vi "STP_22 - three_multiAO+dynamics.vi"() -> ()   [LabVIEW 2010]
uses:
  <vilib>/Math Plots/2D Math Plots/2D Compass/2D Compass XCtrl/2D Compass.xctl
  <vilib>/Platform/TimedLoop/XDataNode/nitl_modes.ctl
  <vilib>/Platform/TimedLoop/XDataNode/XDataNode.xnode
  <vilib>/Platform/TimedLoop/XDataNode/timing_clust.ctl
  <vilib>/Platform/TimedLoop/XDataNode/wakeup.ctl
  <vilib>/Utility/error.llb/DialogType.ctl
  <vilib>/DAQmx/write.llb/DAQmx Write (Analog 1D Wfm NChan NSamp).vi
  <vilib>/DAQmx/write.llb/DAQmx Write (Analog 2D DBL NChan NSamp).vi
  <vilib>/DAQmx/create/timing.llb/DAQmx Create Timing Source (Frequency).vi
  <vilib>/Instr/_visa.llb/VISA Configure Serial Port (Instr).vi
  <vilib>/Math Plots/2D Math Plots/2D Compass/2D Compass Datatype/Public/Plot Helper (Vector).vi
  <vilib>/DAQmx/create/channels.llb/DAQmx Create Channel (AO-Voltage-Basic).vi
  <vilib>/DAQmx/configure/timing.llb/DAQmx Timing (Sample Clock).vi
  <vilib>/daqmx/miscellaneous.llb/DAQmx Fill In Error Info.vi
  <vilib>/measure/matone.llb/Extract Single Tone Information 1 Chan.vi
  <vilib>/measure/NI_MABase.lvlib
  Program Files/National Instruments/LabVIEW 2010/resource/objmgr/daqmx.rc
  <vilib>/Platform/TimedLoop/XDataNode/XDNodeRunTimeDep.lvlib
  <vilib>/measure/NI_MAPro.lvlib
  <vilib>/Math Plots/2D Math Plots/2D Compass/2D Compass Datatype/2D Compass Datatype.lvclass
  <vilib>/Analysis/NI_AALBase.lvlib
  <vilib>/Analysis/NI_AALPro.lvlib
panel:
  out "rocof0":dbl[](array[numeric])
  out "rocof1":dbl[](array[numeric])
  out "ROCOF measured":dbl[](array[numeric])
  out "ROCOF reference":dbl[](array[numeric])
  out "Media":dbl
  in  "stop":bool
  out "Frequency reference":dbl[](array[numeric])
  out "Frequency measured":dbl[](array[numeric])
  out "Angle reference":dbl[](array[numeric])
  out "Angle measured":dbl[](array[numeric])
  out "Voltage reference":dbl[](array[numeric])
  out "Voltage measured":dbl[](array[numeric])
  out "freq1":dbl[](array[numeric])
  out "freq0":dbl[](array[numeric])
  out "magnitude1":dbl[](array[numeric])
  out "magnitude0":dbl[](array[numeric])
  in  "last amp":dbl
  out "phases0":dbl[](array[numeric])
  out "phases1":dbl[](array[numeric])
  out "initialized array":dbl[](array[numeric])
  out "Sine phase":dbl
  in  "Tab Control":T1(tab)
  out "Interf.\nAmplitude (%)":dbl
  out "Interf.\nFrequency (Hz)":dbl
  out "Amplitude (%)":dbl
  out "Harmonic order":i32
  out "reset\nphase?":bool
  out "Samples":dbl
  out "Frequency (Hz)":dbl
  out "Phase (deg)":dbl format="%.4f"
  out "Amplitude (V)":dbl format="%.4g"
  in  "Tab Control 3":T2(tab)
  in  "Interference":bool
  in  "Interf. Frequency":dbl caption="Frequency"
  in  "Interf. Amplitude":dbl caption="Amplitude (%)"
  in  "Amplitude (%)":dbl=10.0
  in  "Order":i32=2
  in  "Harmonics":bool
  in  "phase 2":dbl
  in  "duty cycle (%)":dbl=1.0
  in  "Pulse frequency":dbl=1.0
  in  "Noise":bool
  in  "Amplitude (rms)":dbl=0.0035355 format="%0.6f"
  in  "reset signal":bool
  in  "Phase":dbl format="%#.4f"
  in  "Frequency":dbl=50.0 format="%#.4f"
  in  "Offset":dbl=1.5 format="%#.4f"
  in  "Amplitude":dbl=5.0 format="%#.4f"
  in  "Seconds":dbl=100.0
  in  "Save without\nvariation":bool
  in  "Amp. (%) 4":dbl=10.0 caption="Amplitude (%)"
  in  "Frequency\ninterval 2":dbl=0.25 caption="Frequency\ninterval"
  in  "Final freq. 2":dbl=51.25 caption="Final freq."
  in  "Initial freq. 2":dbl=48.75 caption="Initial freq."
  in  "Interference\nauto variation":bool
  in  "Amp. (%) 3":dbl=10.0 caption="Amplitude (%)"
  in  "Order\ninterval":i32=1
  in  "Final order":i32=50
  in  "Initial order":i32=2
  in  "Harmonics\nauto variation":bool
  in  "Frequency\ninterval":dbl=0.1 format="%.4f"
  in  "Final freq.":dbl=55.0 format="%.4f"
  in  "Initial freq.":dbl=45.0 format="%.4f"
  in  "Freq. auto\nvariation":bool
  in  "Phase\ninterval":dbl=10.0 format="%.4f"
  in  "Final phase":dbl=180.0 format="%.4f"
  in  "Initial phase":dbl=-180.0 format="%.4f"
  in  "Phase auto\nvariation":bool
  in  "Amplitude\ninterval":dbl=0.1 format="%.4f"
  in  "Initial ampl.":dbl=0.5 format="%.4f"
  in  "Final ampl.":dbl=6.0 format="%.4f"
  in  "Ampl. auto\nvariation":bool
  in  "Boolean 2":bool
  in  "Dynamic tests?":bool
  in  "Final fmod":dbl=5.0
  in  "fmod interval":dbl=0.2
  in  "Initial fmod":dbl
  in  "Modulation\nauto variation":bool
  in  "fmod":dbl
  out "fmod (Hz)":dbl
  in  "kx":dbl=0.1
  in  "Enum":T3(ring)
  in  "ka":dbl=0.1
  in  "Freq. Ramp":bool
  in  "Signal generation":bool=TRUE
  in  "File name":path=path "teste.txt"
  in  "Data save":bool
  in  "Boolean":bool
  in  "step time":i32=2
  out "step?":bool
  out "Cycle visualization":dbl[](graph)
  in  "Boolean 3":bool
  out "Phasors visualization":refnum<class "2D Plot Datatype.lvclass">[](xcontrol) caption="2D Compass"
  in  "Porta":refnum<visa-resource-name>="COM5"
  in  "baud rate (kB)":u32=115200
  in  "data bits (8)":u16=8
  in  "timeout (ms)":u32=5000
  in  "parity (0:none)":enum16{"None", "Odd", "Even", "Mark", "Space"}(ring)
  in  "flow control (0:none)":u16(ring) items=["None", "XON/XOFF", "RTS/CTS", "XON/XOFF & RTS/CTS", "DTR/DSR", "XON/XOFF & DTR/DSR"]
  in  "stop bits (10: 1 bit)":u16(ring)=10 items=["1.0"=10, "1.5"=15, "2.0"=20]
  in  "Serial communication":bool=TRUE
  in  "Interference 2":bool caption="Interference"
  in  "amplitude":dbl=1.0 caption="Amp. (%)" format="%#.4p"
  in  "Interf. Frequency 2":dbl=10.0 caption="Frequency (Hz)"
  in  "Harmonics 2":bool caption="Harmonics"
  in  "Amp. (%) 2":dbl caption="Amp. (%)"
  in  "Order 2":i32=2 caption="Order"
  out "Frequency":dbl
  in  "Offset 2":dbl=1.5 caption="Offset"
  out "Phase (degrees) 2":dbl caption="Phase (°)" format="%.4f"
  in  "Amplitude 2":dbl=1.3 caption="Amplitude"
  in  "Frequency 2":dbl=60.0 caption="Frequency"
  in  "Phase 2":dbl caption="Phase"
  in  "reset signal 2":bool caption="reset\nsignal"
  in  "Frequency\noff-set":dbl
  in  "Magnitude\noff-set":dbl
  in  "Magnitude\ncoefficient":dbl=1.0
  in  "Angle\noff-set":dbl
  out "mean rocof":dbl caption="ROCOF (Hz/s)" format="%.8g"
  out "max rocof":dbl caption="ROCOF (Hz/s)" format="%.8g"
  out "mean freq":dbl caption="Frequency (Hz)" format="%.8g"
  out "mean tve":dbl caption="TVE (%)" format="%.8g"
  out "mean phase":dbl caption="Phase (º)" format="%.8g"
  out "mean dev":dbl caption="Magnitude (%)" format="%.8g"
  out "max magnitude":dbl caption="Magnitude (%)" format="%.8g"
  out "max tve":dbl caption="TVE (%)" format="%.8g"
  out "max freq":dbl caption="Frequency (Hz)" format="%.8g"
  out "max phase":dbl caption="Phase (º)" format="%.8g"
  in  "Tab Control 2":T4(tab)
  out "Magnitude measures (V)":dbl[][](graph)
  in  "?":bool
  out "Phase measures (º)":dbl[][](graph)
  in  "?":bool
  in  "Fase ref":enum16{"R", "S", "T"}(ring)
  out "Frequency measures (Hz)":dbl[][](graph)
  in  "?":bool
  out "ROCOF (Hz/s)":dbl[][](graph)
  in  "?":bool
  in  "?":bool
  out "Phase measures (º) 2":dbl[](graph)
  out "Iteration Duration 2":i64
  out "Finished Late? [i-1]":bool
  out "Iteration Duration":i64
  out "Iteration Duration 3":i64
  # "Synchrophasors Test Platform"
  # "A real-time platform for PMU development."
  # "Actual generation"
  # "PPS parameters"
  # "Noise"
  # "Sinusoid parameters"
  # "Max errors:"
  # "Mean errors:"
  # "Signal generation parameters:"
  # "On-line corrections (received data):"
  # "This is a project developed by Flavio Lori Grando, during Masters in Electrical Engineering Graduate Program (PPGEE) of Federal University of Technology - Paraná, Brazil.\n\nContact: flavio.grando.eng@gmail.com"
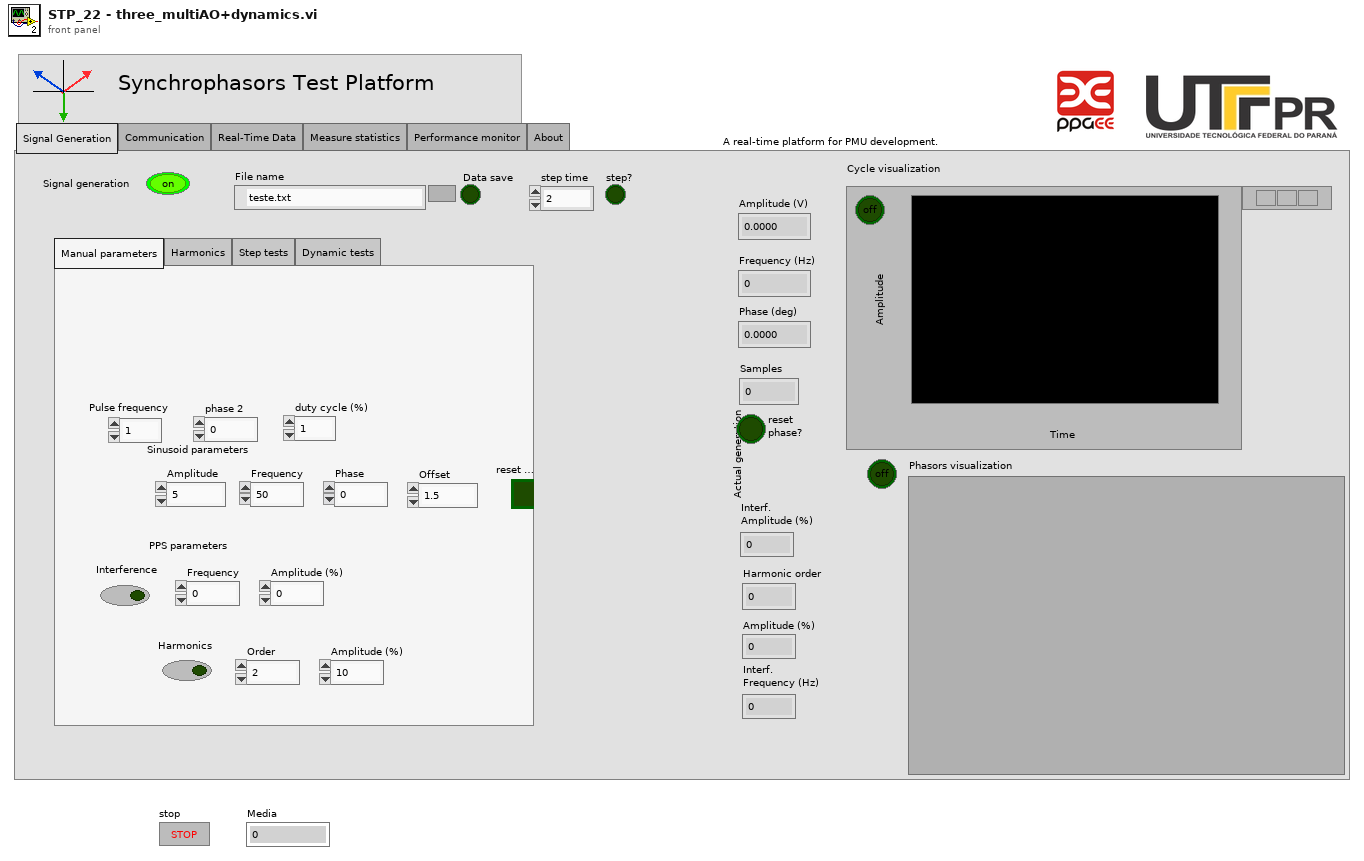
[diagram p1: front panel]
types:
  T1 = enum32{"Signal Generation", "Communication", "Real-Time Data", "Measure statistics", "Performance monitor", "About"}
  T2 = enum32{"Manual parameters", "Harmonics", "Step tests", "Dynamic tests"}
  T3 = enum16{"Amplitude modulation", "Phase modulation", "Frequency ramp", "Frequency ramp 2", "Frequency ramp 3", "Frequency ramp 4", "Frequency ramp 5", "Frequency ramp 6"}
  T4 = enum32{"Magnitude", "Phase", "Frequency", "ROCOF", "Phase deviation"}
  T5 = enum16{"Sine Wave", "Triangle Wave", "Square Wave", "Sawtooth Wave"}
  T6 = typedef "XDNodeRunTimeDep.lvlib/nitl_modes.ctl" = enum32{"No Change", "Process missed periods, maintain original phase", "Discard missed periods, maintain original phase", "Process missed periods, ignore original phase", "Discard missed periods, ignore original phase"}
  T7 = cluster{"frequency":dbl, "amplitude":dbl, "phase":dbl}[]
  T8 = typedef "XDNodeRunTimeDep.lvlib/timing_clust.ctl" = cluster{"Expected End [f-1]":u64, "Actual End [f-1]":u64, "Finished Late? [f-1]":bool, "Expected End [i-1]":u64, "Actual End [i-1]":u64, "Finished Late? [i-1]":bool, "Expected Start [i]":u64, "Actual Start [i]":u64, "Expected Start [f]":u64, "Actual Start [f]":u64, "Source Name":string, "Structure Name":string, "Period":i64, "Deadline":i64, "Offset":i64, "Start":i64, "Priority":i32, "Timeout":i32, "Mode":T6, "Wakeup Reason":T9, "Error":errorcluster, "Source Type":string, "Secondary Source Type":string, "Global End Time":u64, "Global Start Time":u64, "Frame Duration":u64, "Iteration Duration":u64, "Assigned CPU":i32, "I/O Scan Engine Mode":u32}
  T9 = typedef "XDNodeRunTimeDep.lvlib/wakeup.ctl" = enum32{"Normal", "Aborted", "Asynchronous wakeup", "Timing source error", "Timed loop error", "Timeout"}
  T10 = typedef "DialogType.ctl" = u16
  T11 = enum16{"open", "replace", "create", "open or create", "replace or create", "replace or create with confirmation"}
  T12 = cluster{"max ref":dbl, "min ref":dbl, "mean ref":dbl, "max dev":dbl, "min dev":dbl, "mean dev":dbl, "max meas":dbl, "min meas":dbl, "mean meas":dbl}
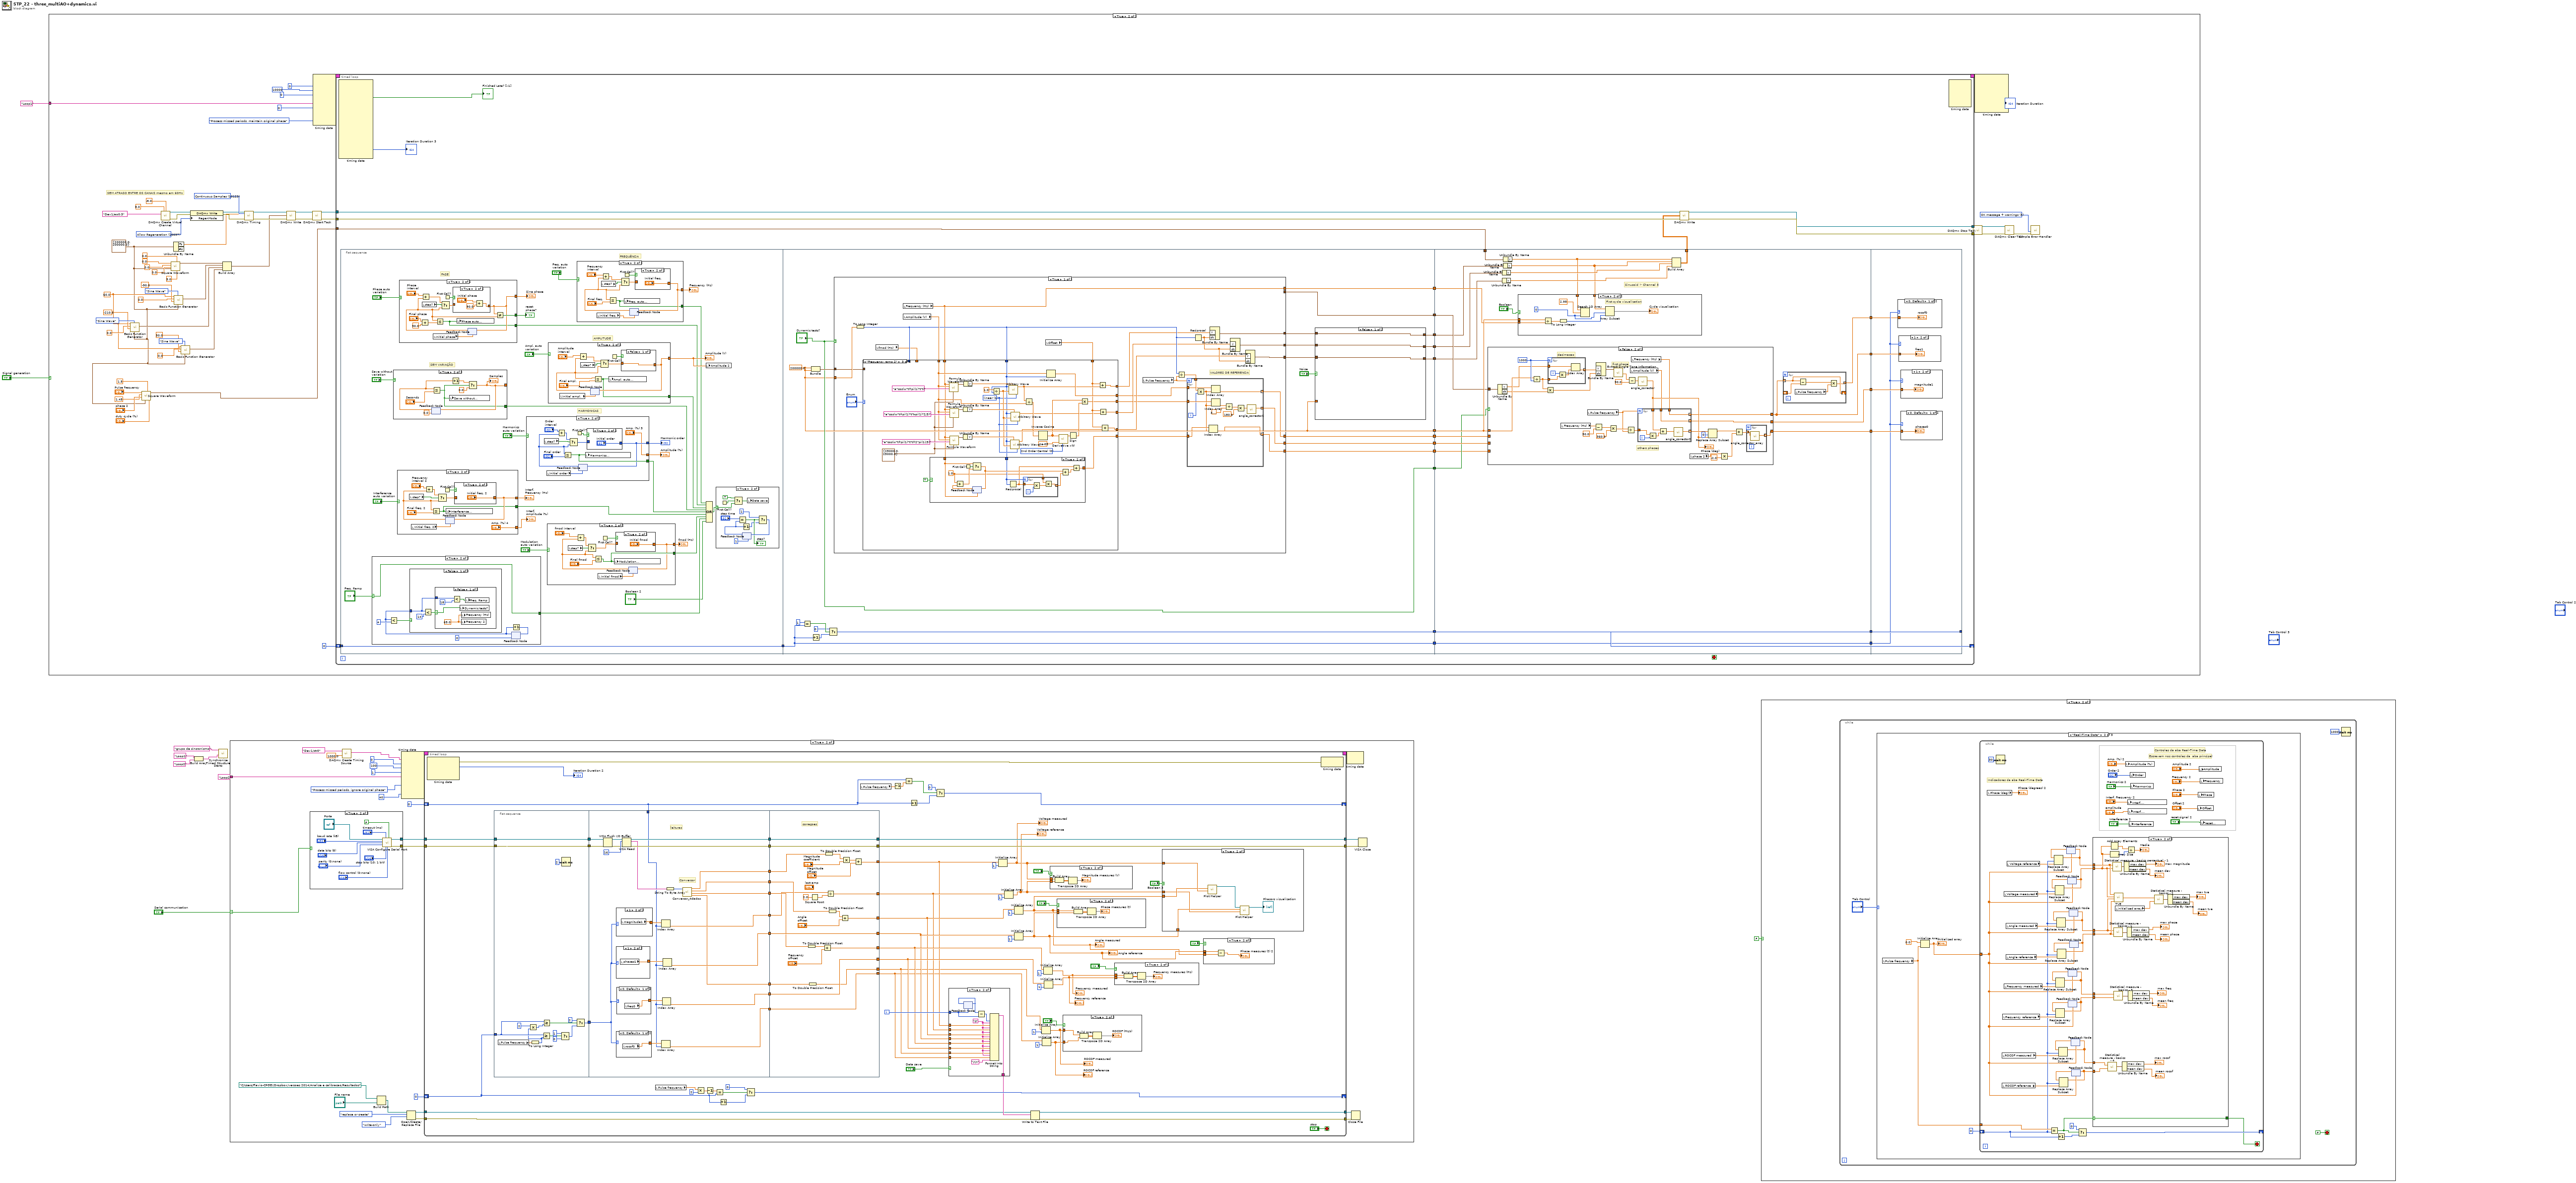
[diagram p0: block diagram]
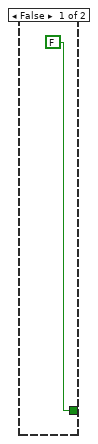
[diagram p4: hidden frame]
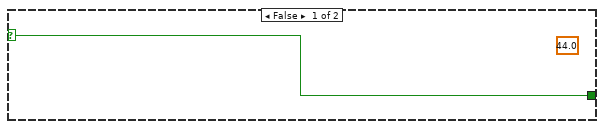
[diagram p7: hidden frame]
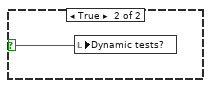
[diagram p8: hidden frame]
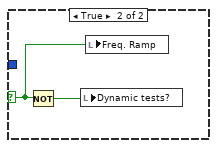
[diagram p9: hidden frame]
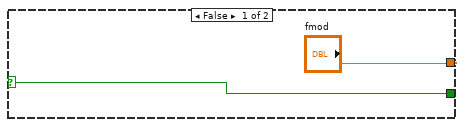
[diagram p10: hidden frame]
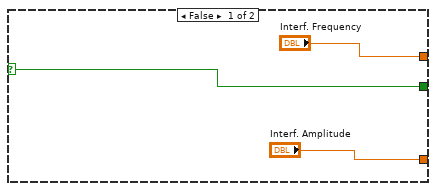
[diagram p12: hidden frame]
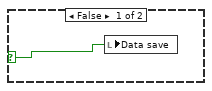
[diagram p14: hidden frame]
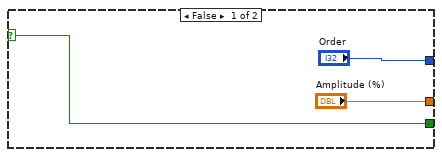
[diagram p15: hidden frame]
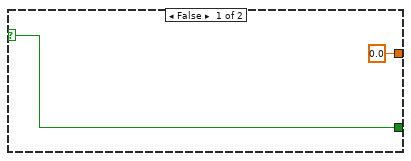
[diagram p17: hidden frame]
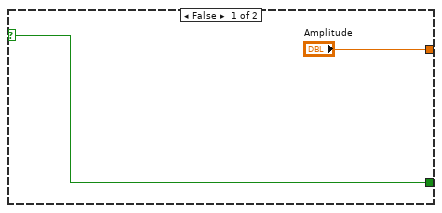
[diagram p18: hidden frame]
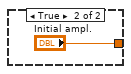
[diagram p19: hidden frame]
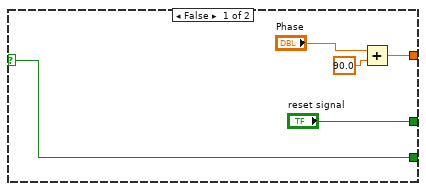
[diagram p20: hidden frame]
diagram:
  n1 = case shown="True" "Signal generation" {
    tunnel: "Loop1" -> [_ w32]
    frame False {
    }
    frame True {
      w19 = 60.0 ("frequency")
      w60 = 10097 items=["Allow Regeneration"=10097, "Do Not Allow Regeneration"=10158] ("RegenMode")
      w13 = cluster{"Fs":dbl, "#s":dbl} {"Fs"=200000.0, "#s"=200000.0} ("Continuous buffer")
      w63 = 10123 items=["Finite Samples"=10178, "Continuous Samples"=10123] ("sample mode")
      w64 = T10 3 items=["no dialog", "OK message", "continue or stop message", "OK message + warnings", "continue/stop + warnings"] ("type of dialog (OK msg:1)")
      # "SEM ATRASO ENTRE OS CANAIS mesmo em 60Hz"
      n2 = call <vilib>:"Basic Function Generator.vi"("sampling info"=w13, "signal type"=T5."Sine Wave" ("signal type 4"), "phase"=-210.0 ("offset 4"), "amplitude"=0.0 ("amplitude 3"), "frequency"=w19) -> ("signal out"=w24:waveform(dbl))  [unwired: 4 in, 2 out]
      n3 = call <vilib>:"Square Waveform.vi"("duty cycle (%)"="duty cycle (%)", "offset"=1.5, "sampling info"=w13, "phase"="phase 2", "amplitude"=1.45, "frequency"="Pulse frequency") -> ("signal out"=w28:waveform(dbl))  [unwired: 4 in, 1 out]
      n4 = call-poly <vilib>:"DAQmx Create Virtual Channel.vi"("maximum value"=8.0 ("Maximum Value"), "minimum value"=-8.0 ("Minimum Value"), "physical channels"=tag "Dev1/ao0:3" ("Physical Channel")) -> ("task out"=w39:refnum<k21>, "error out"=w40:errorcluster)  [unwired: 11 in]
      n5 = call <vilib>:"Square Waveform.vi"("duty cycle (%)"=5.0, "offset"=0.0, "sampling info"=w13, "phase"=0.0, "amplitude"=0.0, "frequency"=0.0) -> ("signal out"=w30:waveform(dbl))  [unwired: 4 in, 1 out]
      n6 = Unbundle By Name(w13) -> ("Fs"=w11:dbl)  [unwired: 1 out]
      n7 = call <vilib>:"Basic Function Generator.vi"("sampling info"=w13, "signal type"=T5."Sine Wave" ("signal type 4"), "phase"=-90.0 ("offset 4"), "amplitude"=0.0 ("amplitude 3"), "frequency"=w19) -> ("signal out"=w31:waveform(dbl))  [unwired: 4 in, 2 out]
      n8 = call <vilib>:"Basic Function Generator.vi"("sampling info"=w13, "signal type"=T5."Sine Wave" ("signal type 4"), "phase"=30.0 ("offset 4"), "amplitude"=0.0 ("amplitude 3"), "frequency"=w19) -> ("signal out"=w20:waveform(dbl))  [unwired: 4 in, 2 out]
      n9 = property class="DAQmx Write"(reference=w39, error in=w40, "RegenMode"=w60) -> (reference out=w12:refnum<k21>, error out=w61:errorcluster)
      n10 = Build Array(w30, w31, w24, w20) -> (w33:waveform(dbl)[])
      n11 = call-poly <vilib>:"DAQmx Timing.vi"("task/channels in"=w12, "sample mode"=w63, "rate"=w11, "error in"=w61) -> ("task out"=w35:refnum<k21>, "error out"=w34:errorcluster)  [unwired: 10 in]
      n12 = call-poly <vilib>:"DAQmx Write.vi"("task/channels in"=w35, "data"=w33, "error in"=w34) -> ("task out"=w44:refnum<k21>, "error out"=w45:errorcluster)  [unwired: 10 in, 1 out]
      n13 = call <vilib>:"DAQmx Start Task.vi"("task/channels in"=w44, "error in"=w45) -> ("task out"=w36:refnum<k21>, "error out"=w37:errorcluster)  [unwired: 12 in]
      n14 = node-c288(i64 0 ("Period"), 10000 ("Priority"), 0 ("Processor"), w32, i64 0 ("Deadline"), nitl_modes."Process missed periods, maintain original phase" ("Mode")) -> (w68:T8)  [unwired: 4 in]
      n15 = timed-loop {
        tunnel: w36 -> [w72]
        tunnel: [w89] -> w53
        tunnel: [w88] -> w52
        timing: w68 -> [_]
        timing-out: [_] -> w67
        shift-right: [w96] -> _
        shift-left: 0 -> [w76]
        tunnel: w37 -> [w90]
        tunnel: w28 -> [w71]
        stop <- _ stop-if-true
        n16 = node-c288() -> (→"Finished Late? [i-1]":bool, →"Iteration Duration 3":i64)  [unwired: 1 in, 15 out]
        n17 = flat-sequence {
          tunnel: w76 -> [w120]
          tunnel: [w120] -> w86
          tunnel: [w275] -> w87
          tunnel: w86 -> [w274]
          tunnel: [w274] -> w85
          tunnel: [w261] -> w84
          tunnel: [w280] -> w83
          tunnel: [w270] -> w81
          tunnel: [w269] -> w80
          tunnel: [w271] -> w79
          tunnel: [w273] -> w78
          tunnel: [w265] -> w75
          tunnel: [w263] -> w74
          tunnel: [w264] -> w73
          tunnel: ["Dynamic tests?"] -> w69
          tunnel: [w679] -> w95
          tunnel: [w677] -> w94
          tunnel: [w670] -> w93
          tunnel: [w658] -> w92
          tunnel: w87 -> [w679]
          tunnel: w85 -> [w678]
          tunnel: [w678] -> w91
          tunnel: [w674] -> w70
          tunnel: w84 -> [w676]
          tunnel: w83 -> [w675]
          tunnel: [w657] -> w82
          tunnel: w81 -> [w669]
          tunnel: w80 -> [w668]
          tunnel: w79 -> [w663]
          tunnel: w78 -> [w673]
          tunnel: w75 -> [w672]
          tunnel: w74 -> [w659]
          tunnel: w73 -> [w671]
          tunnel: w71 -> [w662]
          tunnel: w69 -> [w660]
          tunnel: w95 -> [w749]
          tunnel: [w749] -> w96
          tunnel: w94 -> [w748]
          tunnel: w93 -> [w747]
          tunnel: w92 -> [w746]
          tunnel: w91 -> [w745]
          tunnel: w82 -> [w744]
          frame #0 {
            # "HARMONICAS"
            # "SEM VARIA敲O"
            # "FASE"
            # "FREQUÊNCIA"
            # "AMPLITUDE"
            n18 = case shown="True" "Freq. Ramp" {
              selector: "Freq. Ramp" -> [w126 w127]
              tunnel: [w126 w127] -> w99
              frame False {
                (unwired) 44.0 ("Initial freq. 3")
              }
              frame True {
                n19 = feedback #1(0) -> (w129:i32)
                n20 = Less?(x=w129, y=4) -> (x < y?=w128:bool)
                n21 = case shown="False" w128 {
                  selector: w128 -> [_ w142]
                  tunnel: w129 -> [w134 _]
                  frame False {
                    n22 = Less?(x=w134, y=14) -> (x < y?=w133:bool)
                    n23 = case shown="False" w133 {
                      selector: w133 -> [w136 w141]
                      tunnel: w134 -> [w139 _]
                      frame False {
                        w137 = 65.0 ("Frequency")
                        n24 = Less?(x=w139, y=18) -> (x < y?=w138:bool)
                        n25 = local write "Dynamic tests?"(w136) -> ()
                        n26 = local write "Frequency (Hz)"(w137) -> ()
                        n27 = local write "Frequency 2"(w137) -> ()
                        n28 = local write "Freq. Ramp"(w138) -> ()
                      }
                      frame True {
                        n29 = local write "Dynamic tests?"(w141) -> ()
                      }
                    }
                  }
                  frame True {
                    n30 = Not(x=w142) -> (.not. x?=w143:bool)
                    n31 = local write "Dynamic tests?"(w143) -> ()
                    n32 = local write "Freq. Ramp"(w142) -> ()
                  }
                }
                n33 = Increment(x=w129) -> (x+1=w131:i32)
                n34 = feedback-in #1(w131) -> ()
              }
            }
            n35 = case shown="True" "Save without\nvariation" {
              selector: "Save without\nvariation" -> [w202 _]
              tunnel: [0.0 ("f") w205] -> _
              tunnel: [w202 w204] -> w114
              frame False {
              }
              frame True {
                n36 = feedback #2(0.0 ("f")) -> (w207:dbl)
                n37 = Less Or Equal?(x=w207, y="Seconds") -> (x <= y?=w204:bool)
                n38 = local write "Save without\nvariation"(w204) -> ()
                n39 = Increment(x=w207) -> (x+1=w209:dbl)
                n40 = Select(t=w209, s=w204, f=0.0) -> (s? t:f=w205:dbl)
                "Samples" <- w205
                n41 = feedback-in #2(w205) -> ()
              }
            }
            n42 = case shown="True" "Interference\nauto variation" {
              selector: "Interference\nauto variation" -> [w158 _]
              tunnel: ["Interf. Frequency" w167] -> w106
              tunnel: ["Interf. Amplitude" "Amp. (%) 4"] -> w105
              tunnel: [w158 w161] -> w104
              frame False {
              }
              frame True {
                n43 = local read "step?"() -> (w164:bool)
                n44 = local read "Initial freq. 2"() -> (w168:dbl)
                n45 = First Call?() -> (First Call?: T/F=w171:bool)
                n46 = feedback #3(w168) -> (w163:dbl)
                n47 = Add(x="Frequency\ninterval 2", y=w163) -> (x+y=w165:dbl)
                n48 = Less Or Equal?(x=w163, y="Final freq. 2") -> (x <= y?=w161:bool)
                n49 = Select(t=w165, s=w164, f=w163) -> (s? t:f=w170:dbl)
                n50 = local write "Interference\nauto variation"(w161) -> ()
                n51 = case shown="True" w171 {
                  tunnel: [w172 "Initial freq. 2"] -> w167
                  tunnel: w170 -> [w172 _]
                  frame False {
                  }
                  frame True {
                  }
                }
                n52 = feedback-in #3(w167) -> ()
              }
            }
            "Interf.\nFrequency (Hz)" <- w106
            "Interf.\nAmplitude (%)" <- w105
            n53 = case shown="True" "Phase auto\nvariation" {
              selector: "Phase auto\nvariation" -> [w225 _]
              tunnel: ["reset signal" w240] -> w125
              tunnel: [w227 w239] -> w115
              tunnel: [w225 w234] -> w112
              frame False {
                n54 = Add(x="Phase", y=90.0) -> (x+y=w227:dbl)
              }
              frame True {
                n55 = Add(x="Final phase", y=90.0) -> (x+y=w236:dbl)
                n56 = local read "step?"() -> (w230:bool)
                n57 = local read "Initial phase"() -> (w238:dbl)
                n58 = First Call?() -> (First Call?: T/F=w241:bool)
                n59 = feedback #4(w238) -> (w232:dbl)
                n60 = Add(x="Phase\ninterval", y=w232) -> (x+y=w231:dbl)
                n61 = Less Or Equal?(x=w232, y=w236) -> (x <= y?=w234:bool)
                n62 = Select(t=w231, s=w230, f=w232) -> (s? t:f=w233:dbl)
                n63 = case shown="True" w241 {
                  tunnel: [w243 w244] -> w239
                  tunnel: w233 -> [w243 _]
                  frame False {
                  }
                  frame True {
                    n64 = Add(x="Initial phase", y=90.0) -> (x+y=w244:dbl)
                  }
                }
                n65 = local write "Phase auto\nvariation"(w234) -> ()
                n66 = feedback-in #4(w239) -> ()
                n67 = Not Equal?(x=w239, y=w232) -> (x != y?=w240:bool)
              }
            }
            "Sine phase" <- w115
            "reset\nphase?" <- w125
            n68 = case shown="True" "Harmonics\nauto variation" {
              selector: "Harmonics\nauto variation" -> [w187 _]
              tunnel: ["Order" w193] -> w110
              tunnel: [w187 w194] -> w108
              tunnel: ["Amplitude (%)" "Amp. (%) 3"] -> w109
              frame False {
              }
              frame True {
                n69 = local read "step?"() -> (w196:bool)
                n70 = local read "Initial order"() -> (w198:i32)
                n71 = First Call?() -> (First Call?: T/F=w195:bool)
                n72 = feedback #5(w198) -> (w191:i32)
                n73 = Add(x="Order\ninterval", y=w191) -> (x+y=w190:i32)
                n74 = Less Or Equal?(x=w191, y="Final order") -> (x <= y?=w194:bool)
                n75 = Select(t=w190, s=w196, f=w191) -> (s? t:f=w199:i32)
                n76 = local write "Harmonics\nauto variation"(w194) -> ()
                n77 = case shown="True" w195 {
                  tunnel: [w200 "Initial order"] -> w193
                  tunnel: w199 -> [w200 _]
                  frame False {
                  }
                  frame True {
                  }
                }
                n78 = feedback-in #5(w193) -> ()
              }
            }
            "Harmonic order" <- w110
            "Amplitude (%)" <- w109
            n79 = case shown="True" "Modulation\nauto variation" {
              selector: "Modulation\nauto variation" -> [w145 _]
              tunnel: [w145 w148] -> w102
              tunnel: ["fmod" w147] -> w101
              frame False {
              }
              frame True {
                n80 = local read "step?"() -> (w154:bool)
                n81 = local read "Initial fmod"() -> (w146:dbl)
                n82 = First Call?() -> (First Call?: T/F=w155:bool)
                n83 = feedback #6(w146) -> (w151:dbl)
                n84 = Add(x="fmod interval", y=w151) -> (x+y=w153:dbl)
                n85 = Select(t=w153, s=w154, f=w151) -> (s? t:f=w149:dbl)
                n86 = Less Or Equal?(x=w151, y="Final fmod") -> (x <= y?=w148:bool)
                n87 = local write "Modulation\nauto variation"(w148) -> ()
                n88 = case shown="True" w155 {
                  tunnel: [w156 "Initial fmod"] -> w147
                  tunnel: w149 -> [w156 _]
                  frame False {
                  }
                  frame True {
                  }
                }
                n89 = feedback-in #6(w147) -> ()
              }
            }
            "fmod (Hz)" <- w101
            n90 = case shown="True" "Ampl. auto\nvariation" {
              selector: "Ampl. auto\nvariation" -> [w211 _]
              tunnel: ["Amplitude" w220] -> w119
              tunnel: [w211 w215] -> w113
              frame False {
              }
              frame True {
                n91 = local read "Initial ampl."() -> (w219:dbl)
                n92 = local read "step?"() -> (w216:bool)
                n93 = feedback #7(w219) -> (w214:dbl)
                n94 = Add(x="Amplitude\ninterval", y=w214) -> (x+y=w218:dbl)
                n95 = Less Or Equal?(x=w214, y="Final ampl.") -> (x <= y?=w215:bool)
                n96 = Select(t=w218, s=w216, f=w214) -> (s? t:f=w217:dbl)
                n97 = local write "Ampl. auto\nvariation"(w215) -> ()
                n98 = First Call?() -> (First Call?: T/F=w221:bool)
                n99 = case shown="False" w221 {
                  tunnel: [w223 "Initial ampl."] -> w220
                  tunnel: w217 -> [w223 _]
                  frame False {
                  }
                  frame True {
                  }
                }
                n100 = feedback-in #7(w220) -> ()
              }
            }
            "Amplitude (V)" <- w119
            n101 = case shown="True" "Freq. auto\nvariation" {
              selector: "Freq. auto\nvariation" -> [w248 _]
              tunnel: ["Frequency" w255] -> w117
              tunnel: [w248 w253] -> w111
              frame False {
              }
              frame True {
                n102 = local read "Initial freq."() -> (w254:dbl)
                n103 = local read "step?"() -> (w249:bool)
                n104 = First Call?() -> (First Call?: T/F=w257:bool)
                n105 = feedback #8(w254) -> (w250:dbl)
                n106 = Add(x="Frequency\ninterval", y=w250) -> (x+y=w251:dbl)
                n107 = Less Or Equal?(x=w250, y="Final freq.") -> (x <= y?=w253:bool)
                n108 = Select(t=w251, s=w249, f=w250) -> (s? t:f=w252:dbl)
                n109 = local write "Freq. auto\nvariation"(w253) -> ()
                n110 = case shown="True" w257 {
                  tunnel: [w259 "Initial freq."] -> w255
                  tunnel: w252 -> [w259 _]
                  frame False {
                  }
                  frame True {
                  }
                }
                n111 = feedback-in #8(w255) -> ()
              }
            }
            "Frequency (Hz)" <- w117
            n112 = local write "Amplitude 2"(w119) -> ()
            n113 = Compound Arithmetic op=OR(w111, w112, w113, w114, w108, w104, w102, w99, "Boolean 2") -> (w116:bool)
            n114 = case shown="True" w116 {
              selector: w116 -> [w174 w183]
              frame False {
                n115 = local write "Data save"(w174) -> ()
              }
              frame True {
                n116 = First Call?() -> (First Call?: T/F=w185:bool)
                n117 = Select(t=TRUE, s=w185, f=w183) -> (s? t:f=w182:bool)
                n118 = feedback #9(1 ("f")) -> (w175:i32)
                n119 = Equal?(x="step time", y=w175) -> (x = y?=w178:bool)
                "step?" <- w178
                n120 = Increment(x=w175) -> (x+1=w176:i32)
                n121 = local write "Data save"(w182) -> ()
                n122 = Select(t=1 ("f"), s=w178, f=w176) -> (s? t:f=w181:i32)
                n123 = feedback-in #9(w181) -> ()
              }
            }
          }
          frame #1 {
            w261 = 200000.0 ("#s")
            n124 = Equal?(x=1, y=w274) -> (x = y?=w279:bool)
            n125 = Bundle("#s"=w261, "#s"=w261) -> (w281:cluster{"#s":dbl, "#s":dbl})  [unwired: 1 in]
            n126 = Increment(x=w274) -> (x+1=w277:i32)
            n127 = Select(t=0, s=w279, f=w277) -> (s? t:f=w275:i32)
            n128 = case shown="True" "Dynamic tests?" {
              tunnel: w281 -> [w305 w601]
              tunnel: [w309 w603] -> w280
              tunnel: [w314 w595] -> w272
              tunnel: [w313 w594] -> w268
              tunnel: [w319 w590] -> w266
              tunnel: [_ w585] -> w273
              tunnel: w261 -> [w317 _]
              tunnel: [w308 _] -> w265
              tunnel: [w307 _] -> w264
              tunnel: [w298 _] -> w263
              frame True {
                # "VALORES DE REFERENCIA"
                n129 = To Long Integer(number=w317) -> (32bit integer=w311:i32)
                n130 = local read "fmod (Hz)"() -> (w306:dbl)
                n131 = local read "Frequency (Hz)"() -> (w309:dbl)
                n132 = local read "Amplitude (V)"() -> (w318:dbl)
                n133 = local read "Offset"() -> (w297:dbl)
                n134 = case shown="\"Frequency ramp 2\"" "Enum" {
                  tunnel: w318 -> [w331 w367 w425 w487 w500 _ w512 w559]
                  tunnel: w309 -> [w328 _ w423 w478 _ _ w514 w545]
                  tunnel: w311 -> [_ w374 w428 _ _ _ w513 w538]
                  tunnel: [w345 w381 w414 w481 _ _ w506 w554] -> w299
                  tunnel: [w325 w382 w420 w488 w498 _ w504 w536] -> w302
                  tunnel: [w323 w380 w415 w488 w497 _ w523 w547] -> w304
                  tunnel: [w322 w379 w417 w488 w496 _ w522 w546] -> w303
                  tunnel: w311 -> [w327 w375 _ w485 w495 _ _ w534]
                  tunnel: [w339 w372 w427 w483 _ _ w503 w544] -> w300
                  tunnel: w306 -> [w337 _ _ _ _ _ _ w539]
                  tunnel: w305 -> [w338 _ _ w489 _ _ _ w537]
                  tunnel: [w330 _ w431 _ _ _ w511 w536] -> w301
                  tunnel: w297 -> [w321 _ w419 _ _ _ _ _]
                  frame "Phase modulation" {
                    # "referencia"
                    n135 = call <vilib>:"Sine Waveform.vi"("sampling info"=w338, "phase"=-90.0, "amplitude"="ka", "frequency"=w337) -> ("signal out"=w341:waveform(dbl))  [unwired: 6 in, 1 out]
                    n136 = call <vilib>:"Sine Waveform.vi"("sampling info"=w338, "phase"=-180.0, "amplitude"="ka", "frequency"=w337) -> ("signal out"=w335:waveform(dbl))  [unwired: 6 in, 1 out]
                    n137 = Unbundle By Name(w341) -> ("Y"=w332:dbl[])
                    n138 = Unbundle By Name(w335) -> ("Y"=w334:dbl[])
                    n139 = Reciprocal(x=w327) -> (1/x=w329:dbl)
                    n140 = Multiply(x=w328, y=6.283185307179586) -> (x*y=w343:dbl)
                    n141 = Divide(x=6.283185307179586, y=3.0) -> (x/y=w348:dbl)
                    n142 = Multiply(x=w343, y=w329) -> (x*y=w344:dbl)
                    n143 = for {
                      N: w327 -> [_]
                      tunnel: w344 -> [w356]
                      tunnel: [w364] -> w351 mode=indexing
                      tunnel: [w353] -> w345 mode=indexing
                      tunnel: w348 -> [w361]
                      tunnel: [w360] -> w347 mode=indexing
                      tunnel: [w359] -> w346 mode=indexing
                      tunnel: w332 -> [w353] mode=indexing
                      tunnel: [w354] -> w330 mode=indexing
                      tunnel: w331 -> [w354]
                      i -> [w355]
                      n144 = Multiply(x=w356, y=w355) -> (x*y=w358:dbl)
                      n145 = Add(x=w358, y=w353) -> (x+y=w357:dbl)
                      n146 = Add(x=w357, y=w361) -> (x+y=w362:dbl)
                      n147 = Subtract(x=w357, y=w361) -> (x-y=w363:dbl)
                      n148 = Cosine(x=w362) -> (cos(x)=w360:dbl)
                      n149 = Cosine(x=w363) -> (cos(x)=w359:dbl)
                      n150 = Cosine(x=w357) -> (cos(x)=w364:dbl)
                    }
                    n151 = Multiply(x=w334, y=w337) -> (x*y=w340:dbl[])
                    n152 = Multiply(x=w331, y=w346) -> (x*y=w324:dbl[])
                    n153 = Multiply(x=w331, y=w347) -> (x*y=w320:dbl[])
                    n154 = Multiply(x=w331, y=w351) -> (x*y=w326:dbl[])
                    n155 = Subtract(x=w328, y=w340) -> (x-y=w339:dbl[])
                    n156 = Add(x=w321, y=w326) -> (x+y=w325:dbl[])
                    n157 = Add(x=w321, y=w320) -> (x+y=w322:dbl[])
                    n158 = Add(x=w321, y=w324) -> (x+y=w323:dbl[])
                  }
                  frame "Frequency ramp" {
                    w366 = 6.283185307179586
                    n159 = Bundle("#s"=50000.0, "#s"=500000.0) -> (w370:cluster{"#s":dbl, "#s":dbl})  [unwired: 1 in]
                    n160 = case shown="False" FALSE {
                      tunnel: [w397 w401] -> w368
                      tunnel: w375 -> [w393 _]
                      tunnel: w370 -> [_ w399]
                      frame False {
                        n161 = Divide(x=0.5 ("samples"), y=w393) -> (x/y=w396:dbl)
                        n162 = call <vilib>:"Sawtooth Wave.vi"("samples"=w393, "frequency"=w396, "reset phase"=FALSE) -> ("sawtooth wave"=w394:dbl[])  [unwired: 2 in, 2 out]
                        n163 = Negate(x=w394) -> (-x=w397:dbl[])
                      }
                      frame True {
                        n164 = call <vilib>:"Sawtooth Waveform.vi"("sampling info"=w399, "reset signal"=TRUE, "frequency"=0.5) -> ("signal out"=w402:waveform(dbl))  [unwired: 7 in, 1 out]
                        n165 = Unbundle By Name(w402) -> ("Y"=w401:dbl[])
                      }
                    }
                    n166 = Multiply(x=w366, y=w366) -> (x*y=w390:dbl)
                    n167 = Multiply(x=w368, y=3.141592653589793) -> (x*y=w377:dbl[])
                    n168 = Divide(x=6.283185307179586, y=3.0) -> (x/y=w385:dbl)
                    n169 = Multiply(x=w390, y=1e-05) -> (x*y=w389:dbl)
                    n170 = Multiply(x=w377, y=1e-05) -> (x*y=w376:dbl[])
                    n171 = for {
                      N: w374 -> [_]
                      tunnel: w389 -> [w405]
                      tunnel: [w412] -> w388 mode=indexing
                      tunnel: [w406] -> w381 mode=indexing
                      tunnel: w385 -> [w409]
                      tunnel: [w408] -> w384 mode=indexing
                      tunnel: [w407] -> w383 mode=indexing
                      tunnel: w376 -> [w404] mode=indexing
                      i -> [w413]
                      n172 = Add(x=w405, y=w404) -> (x+y=w403:dbl)
                      n173 = Multiply(x=w403, y=w413) -> (x*y=w406:dbl)
                      n174 = Add(x=w406, y=w409) -> (x+y=w410:dbl)
                      n175 = Subtract(x=w406, y=w409) -> (x-y=w411:dbl)
                      n176 = Cosine(x=w410) -> (cos(x)=w408:dbl)
                      n177 = Cosine(x=w411) -> (cos(x)=w407:dbl)
                      n178 = Cosine(x=w406) -> (cos(x)=w412:dbl)
                    }
                    n179 = Multiply(x=w367, y=w383) -> (x*y=w380:dbl[])
                    n180 = Multiply(x=w367, y=w384) -> (x*y=w379:dbl[])
                    n181 = Multiply(x=w367, y=w388) -> (x*y=w382:dbl[])
                    n182 = Add(x=w368, y=w368) -> (x+y=w372:dbl[])
                  }
                  frame "Frequency ramp 2" {
                    w434 = u16 0 items=["2nd Order Central", "4th Order Central", "Forward", "Backward"] ("method")
                    w429 = 1 items=["none", "linear"] ("interpolation")
                    w440 = cluster{"Fs":dbl, "#s":dbl} {"Fs"=25000.0, "#s"=25000.0} ("sampling info")
                    n183 = case shown="True" TRUE {
                      tunnel: w428 -> [w450 w468]
                      tunnel: [w447 w465] -> w427
                      tunnel: w423 -> [w451 w463]
                      frame False {
                        n184 = First Call?() -> (First Call?: T/F=w453:bool)
                        n185 = feedback #10(w451) -> (w454:dbl)
                        n186 = Decrement(x=w454) -> (x-1=w452:dbl)
                        n187 = Select(t=w451, s=w453, f=w452) -> (s? t:f=w455:dbl)
                        n188 = feedback-in #10(w455) -> ()
                        n189 = Reciprocal(x=w450) -> (1/x=w448:dbl)
                        n190 = for {
                          N: w450 -> [_]
                          tunnel: w448 -> [w459]
                          tunnel: [w458] -> w456 mode=indexing
                          i -> [w457]
                          n191 = Multiply(x=w459, y=w457) -> (x*y=w458:dbl)
                        }
                        n192 = Subtract(x=w455, y=w456) -> (x-y=w449:dbl[])
                        n193 = Subtract(x=w449, y=w448) -> (x-y=w447:dbl[])
                      }
                      frame True {
                        w460 = 1.0 ("x")
                        n194 = First Call?() -> (First Call?: T/F=w470:bool)
                        n195 = feedback #11(w463) -> (w462:dbl)
                        n196 = Add(x=w460, y=w462) -> (x+y=w461:dbl)
                        n197 = Select(t=w463, s=w470, f=w461) -> (s? t:f=w469:dbl)
                        n198 = feedback-in #11(w469) -> ()
                        n199 = Reciprocal(x=w468) -> (1/x=w464:dbl)
                        n200 = for {
                          N: w468 -> [_]
                          tunnel: w464 -> [w475]
                          tunnel: [w472] -> w467 mode=indexing
                          tunnel: w460 -> [w471]
                          i -> [w474]
                          n201 = Multiply(x=w475, y=w474) -> (x*y=w473:dbl)
                          n202 = Multiply(x=w471, y=w473) -> (x*y=w472:dbl)
                        }
                        n203 = Add(x=w469, y=w467) -> (x+y=w466:dbl[])
                        n204 = Add(x=w464, y=w466) -> (x+y=w465:dbl[])
                      }
                    }
                    n205 = call <vilib>:"Formula Waveform.vi"("sampling info"=w440, "formula"="a*cos(w*t+pi(1)*t*t)", "amplitude"=w425, "frequency"=w423) -> ("signal out"=w445:waveform(dbl))  [unwired: 6 in, 1 out]
                    n206 = call <vilib>:"Formula Waveform.vi"("sampling info"=w440, "formula"="a*cos(w*t+pi(1)*t*t-pi(1)*2/3)", "amplitude"=w425, "frequency"=w423) -> ("signal out"=w442:waveform(dbl))  [unwired: 6 in, 1 out]
                    n207 = call <vilib>:"Formula Waveform.vi"("sampling info"=w440, "formula"="a*cos(w*t+pi(1)*t*t+2*pi(1)/3)", "amplitude"=w425, "frequency"=w423) -> ("signal out"=w441:waveform(dbl))  [unwired: 6 in, 1 out]
                    n208 = Unbundle By Name(w442) -> ("Y"=w437:dbl[])
                    n209 = Unbundle By Name(w441) -> ("Y"=w436:dbl[])
                    n210 = Unbundle By Name(w445) -> ("Y"=w438:dbl[])
                    n211 = Divide(x=1.0, y=w428) -> (x/y=w435:dbl)
                    n212 = call <vilib>:"Arbitrary Wave.vi"("interpolation"=w429, "Wave Table"=w438, "frequency"=w435, "samples"=w428) -> ("arbitrary wave"=w421:dbl[])  [unwired: 3 in, 2 out]
                    n213 = call <vilib>:"Arbitrary Wave.vi"("interpolation"=w429, "Wave Table"=w436, "frequency"=w435, "samples"=w428) -> ("arbitrary wave"=w418:dbl[])  [unwired: 3 in, 2 out]
                    n214 = call <vilib>:"Arbitrary Wave.vi"("interpolation"=w429, "Wave Table"=w437, "frequency"=w435, "samples"=w428) -> ("arbitrary wave"=w416:dbl[])  [unwired: 3 in, 2 out]
                    n215 = Divide(x=w421, y=w425) -> (x/y=w424:dbl[])
                    n216 = Inverse Cosine(1:w424) -> (0:w426:dbl[])
                    n217 = Initialize Array(w425, w428) -> (w431:dbl[])
                    n218 = call <vilib>:"Derivative x(t).vi"("method"=w434, "dt"=1e-05, "X"=w426) -> ("dX/dt"=w432:dbl[])  [unwired: 7 in, 1 out]
                    n219 = Sign(1:w432) -> (0:w430:dbl[])
                    n220 = Multiply(x=w426, y=w430) -> (x*y=w414:dbl[])
                    n221 = Add(x=w419, y=w421) -> (x+y=w420:dbl[])
                    n222 = Add(x=w419, y=w416) -> (x+y=w415:dbl[])
                    n223 = Add(x=w419, y=w418) -> (x+y=w417:dbl[])
                  }
                  frame "Frequency ramp 3" {
                    n224 = Reciprocal(x=w485) -> (1/x=w486:dbl)
                    n225 = for {
                      N: w485 -> [_]
                      tunnel: w486 -> [w494]
                      tunnel: [w492] -> w484 mode=indexing
                      i -> [w493]
                      n226 = Multiply(x=w494, y=w493) -> (x*y=w492:dbl)
                    }
                    n227 = First Call?() -> (First Call?: T/F=w479:bool)
                    n228 = call <vilib>:"Formula Waveform.vi"("sampling info"=w489, "formula"="a*cos(w*t+pi(1)*t*t)", "amplitude"=w487, "frequency"=w478) -> ("signal out"=w490:waveform(dbl))  [unwired: 6 in, 1 out]
                    n229 = feedback #12(w478) -> (w476:dbl)
                    n230 = Increment(x=w476) -> (x+1=w480:dbl)
                    n231 = Select(t=w478, s=w479, f=w480) -> (s? t:f=w477:dbl)
                    n232 = feedback-in #12(w477) -> ()
                    n233 = Unbundle By Name(w490) -> ("Y"=w488:dbl[])
                    n234 = Add(x=w477, y=w484) -> (x+y=w483:dbl[])
                    n235 = Divide(x=w488, y=w487) -> (x/y=w482:dbl[])
                    n236 = Inverse Cosine(1:w482) -> (0:w481:dbl[])
                  }
                  frame "Frequency ramp 4" {
                    w501 = 1 items=["none", "linear"] ("interpolation")
                    n237 = Divide(x=1.0, y=w495) -> (x/y=w499:dbl)
                    n238 = call <vilib>:"Arbitrary Wave.vi"("interpolation"=w501, "frequency"=w499, "amplitude"=w500, "samples"=w495) -> ("arbitrary wave"=w497:dbl[])  [unwired: 3 in, 2 out]
                    n239 = call <vilib>:"Arbitrary Wave.vi"("interpolation"=w501, "frequency"=w499, "amplitude"=w500, "samples"=w495) -> ("arbitrary wave"=w498:dbl[])  [unwired: 3 in, 2 out]
                    n240 = call <vilib>:"Arbitrary Wave.vi"("interpolation"=w501, "frequency"=w499, "amplitude"=w500, "samples"=w495) -> ("arbitrary wave"=w496:dbl[])  [unwired: 3 in, 2 out]
                  }
                  frame "Frequency ramp 5" {
                  }
                  frame "Frequency ramp 6" {
                    w510 = u16 3 items=["2nd Order Central", "4th Order Central", "Forward", "Backward"] ("method")
                    w524 = cluster{"Fs":dbl, "#s":dbl} {"Fs"=25000.0, "#s"=25000.0} ("sampling info")
                    n241 = call <vilib>:"Formula Waveform.vi"("sampling info"=w524, "formula"="a*cos(w*t+pi(1)*t*t)", "amplitude"=w512, "frequency"=w514) -> ("signal out"=w529:waveform(dbl))  [unwired: 6 in, 1 out]
                    n242 = call <vilib>:"Formula Waveform.vi"("sampling info"=w524, "formula"="a*cos(w*t+pi(1)*t*t-pi(1)*2/3)", "amplitude"=w512, "frequency"=w514) -> ("signal out"=w526:waveform(dbl))  [unwired: 6 in, 1 out]
                    n243 = call <vilib>:"Formula Waveform.vi"("sampling info"=w524, "formula"="a*cos(w*t+pi(1)*t*t+2*pi(1)/3)", "amplitude"=w512, "frequency"=w514) -> ("signal out"=w525:waveform(dbl))  [unwired: 6 in, 1 out]
                    n244 = Unbundle By Name(w526) -> ("Y"=w523:dbl[])
                    n245 = Unbundle By Name(w525) -> ("Y"=w522:dbl[])
                    n246 = Unbundle By Name(w529) -> ("Y"=w504:dbl[])
                    n247 = First Call?() -> (First Call?: T/F=w520:bool)
                    n248 = feedback #13(w514) -> (w519:dbl)
                    n249 = Increment(x=w519) -> (x+1=w521:dbl)
                    n250 = Select(t=w514, s=w520, f=w521) -> (s? t:f=w518:dbl)
                    n251 = feedback-in #13(w518) -> ()
                    n252 = Reciprocal(x=w513) -> (1/x=w515:dbl)
                    n253 = for {
                      N: w513 -> [_]
                      tunnel: w515 -> [w533]
                      tunnel: [w532] -> w517 mode=indexing
                      i -> [w531]
                      n254 = Multiply(x=w533, y=w531) -> (x*y=w532:dbl)
                    }
                    n255 = Inverse Cosine(1:w504) -> (0:w505:dbl[])
                    n256 = call <vilib>:"Derivative x(t).vi"("method"=w510, "dt"=1e-05, "X"=w505) -> ("dX/dt"=w508:dbl[])  [unwired: 7 in, 1 out]
                    n257 = Sign(1:w508) -> (0:w507:dbl[])
                    n258 = Add(x=w518, y=w517) -> (x+y=w516:dbl[])
                    n259 = Initialize Array(w512, w513) -> (w511:dbl[])
                    n260 = Add(x=w515, y=w516) -> (x+y=w503:dbl[])
                    n261 = Multiply(x=w505, y=w507) -> (x*y=w506:dbl[])
                  }
                  frame "Amplitude modulation" {
                    n262 = call <vilib>:"Sine Waveform.vi"("sampling info"=w537, "phase"=90.0 ("phase in"), "amplitude"="kx", "frequency"=w539) -> ("signal out"=w541:waveform(dbl))  [unwired: 6 in, 1 out]
                    n263 = Unbundle By Name(w541) -> ("Y"=w540:dbl[])
                    n264 = Add(x=w559, y=w540) -> (x+y=w548:dbl[])
                    n265 = Reciprocal(x=w534) -> (1/x=w535:dbl)
                    n266 = Multiply(x=w545, y=6.283185307179586) -> (x*y=w557:dbl)
                    n267 = Divide(x=6.283185307179586, y=3.0) -> (x/y=w551:dbl)
                    n268 = Multiply(x=w557, y=w535) -> (x*y=w556:dbl)
                    n269 = for {
                      N: w538 -> [_]
                      tunnel: w556 -> [w567]
                      tunnel: [w568] -> w555 mode=indexing
                      tunnel: [w564] -> w554 mode=indexing
                      tunnel: w551 -> [w563]
                      tunnel: [w562] -> w550 mode=indexing
                      tunnel: [w561] -> w549 mode=indexing
                      tunnel: [w560] -> w544 mode=indexing
                      tunnel: w545 -> [w560]
                      i -> [w569]
                      n270 = Multiply(x=w567, y=w569) -> (x*y=w564:dbl)
                      n271 = Add(x=w564, y=w563) -> (x+y=w565:dbl)
                      n272 = Subtract(x=w564, y=w563) -> (x-y=w566:dbl)
                      n273 = Cosine(x=w565) -> (cos(x)=w562:dbl)
                      n274 = Cosine(x=w566) -> (cos(x)=w561:dbl)
                      n275 = Cosine(x=w564) -> (cos(x)=w568:dbl)
                    }
                    n276 = Multiply(x=w548, y=w549) -> (x*y=w547:dbl[])
                    n277 = Multiply(x=w548, y=w550) -> (x*y=w546:dbl[])
                    n278 = Multiply(x=w548, y=w555) -> (x*y=w536:dbl[])
                  }
                }
                n279 = local read "Pulse frequency"() -> (w316:dbl)
                n280 = Divide(x=w311, y=w316) -> (x/y=w315:dbl)
                n281 = for {
                  N: w316 -> [_]
                  tunnel: w299 -> [w583]
                  tunnel: w315 -> [w581]
                  tunnel: [w574] -> w308 mode=indexing
                  tunnel: w301 -> [w575]
                  tunnel: [w573] -> w307 mode=indexing
                  tunnel: w300 -> [w572]
                  tunnel: [w570] -> w298 mode=indexing
                  i -> [w582]
                  n282 = Multiply(x=w581, y=w582) -> (x*y=w571:dbl)
                  n283 = Index Array(array=w572, index=w571) -> (element=w570:dbl)
                  n284 = Index Array(array=w583, index=w571) -> (element=w578:dbl)
                  n285 = Index Array(array=w575, index=w571) -> (element=w574:dbl)
                  n286 = Divide(x=w578, y=3.141592653589793) -> (x/y=w577:dbl)
                  n287 = Multiply(x=w577, y=180.0) -> (x*y=w576:dbl)
                  n288 = call "angle_corrector2.vi"("angle"=w576) -> ("angle corrected"=w573:dbl)  [unwired: 10 in]
                }
                n289 = Reciprocal(x=w311) -> (1/x=w312:dbl)
                n290 = Bundle By Name("Y"=w302, "dt"=w312) -> (w319:waveform(dbl))  [unwired: 1 in]
                n291 = Bundle By Name("Y"=w304, "dt"=w312) -> (w314:waveform(dbl))  [unwired: 1 in]
                n292 = Bundle By Name("Y"=w303, "dt"=w312) -> (w313:waveform(dbl))  [unwired: 1 in]
              }
              frame False {
                # "Sinusoid configurations"
                n293 = local read "reset\nphase?"() -> (w602:bool)
                n294 = local read "Frequency (Hz)"() -> (w603:dbl)
                n295 = local read "Amplitude (V)"() -> (w604:dbl)
                n296 = local read "Sine phase"() -> (w608:dbl)
                n297 = local write "Offset 2"("Offset") -> ()
                n298 = Subtract(x=w608, y=120.0) -> (x-y=w610:dbl)
                n299 = call <vilib>:"Sine Waveform.vi"("offset"="Offset", "sampling info"=w601, "reset signal"=w602, "phase"=w608, "amplitude"=w604, "frequency"=w603) -> ("signal out"=w588:waveform(dbl))  [unwired: 4 in, 1 out]
                n300 = Subtract(x=w608, y=240.0) -> (x-y=w607:dbl)
                n301 = call <vilib>:"Sine Waveform.vi"("offset"="Offset", "sampling info"=w601, "reset signal"=w602, "phase"=w610, "amplitude"=w604, "frequency"=w603) -> ("signal out"=w587:waveform(dbl))  [unwired: 4 in, 1 out]
                n302 = call <vilib>:"Sine Waveform.vi"("offset"="Offset", "sampling info"=w601, "reset signal"=w602, "phase"=w607, "amplitude"=w604, "frequency"=w603) -> ("signal out"=w586:waveform(dbl))  [unwired: 4 in, 1 out]
                n303 = case shown="\"R\"" "Fase ref" {
                  tunnel: w588 -> [_ _ w615]
                  tunnel: w587 -> [w613 _ _]
                  tunnel: w586 -> [_ w614 _]
                  tunnel: [w613 w614 w615] -> w585
                  frame "S" {
                  }
                  frame "T" {
                  }
                  frame "R" {
                  }
                }
                n304 = local read "Harmonics\nauto variation"() -> (w597:bool)
                n305 = local read "Amplitude (V)"() -> (w596:dbl)
                n306 = Or(x=w597, y="Harmonics") -> (x .or. y?=w599:bool)
                n307 = case shown="True" w599 {
                  tunnel: w586 -> [w638 w651]
                  tunnel: [w638 w650] -> w612
                  tunnel: w601 -> [_ w649]
                  tunnel: w587 -> [w637 w647]
                  tunnel: w588 -> [w636 w646]
                  tunnel: [w637 w644] -> w606
                  tunnel: [w636 w643] -> w605
                  tunnel: [w635 w640] -> w600
                  tunnel: w596 -> [w635 w640]
                  frame False {
                  }
                  frame True {
                    n308 = local read "Amplitude (%)"() -> (w642:dbl)
                    n309 = local read "Harmonic order"() -> (w648:i32)
                    n310 = local read "Frequency (Hz)"() -> (w641:dbl)
                    n311 = Divide(x=w642, y=100.0) -> (x/y=w653:dbl)
                    n312 = Multiply(x=w641, y=w648) -> (x*y=w656:dbl)
                    "Frequency" <- w656
                    n313 = Multiply(x=w640, y=w653) -> (x*y=w652:dbl)
                    n314 = call <vilib>:"Sine Waveform.vi"("sampling info"=w649, "phase"=0.0, "amplitude"=w652, "frequency"=w656) -> ("error out"=w639:errorcluster, "signal out"=w645:waveform(dbl))  [unwired: 6 in]
                    n315 = Add(1:w645, 2:w646, 4:w639) -> (0:w643:waveform(dbl))  [unwired: 1 out]
                    n316 = Add(1:w645, 2:w647, 4:w639) -> (0:w644:waveform(dbl))  [unwired: 1 out]
                    n317 = Add(1:w645, 2:w651, 4:w639) -> (0:w650:waveform(dbl))  [unwired: 1 out]
                  }
                }
                n318 = local read "Interference\nauto variation"() -> (w591:bool)
                n319 = Or(x="Interference", y=w591) -> (x .or. y?=w593:bool)
                n320 = case shown="True" w593 {
                  tunnel: w600 -> [_ w631]
                  tunnel: w601 -> [_ w630]
                  tunnel: w612 -> [w618 w629]
                  tunnel: [w618 w628] -> w594
                  tunnel: w606 -> [w617 w627]
                  tunnel: w605 -> [w616 w625]
                  tunnel: [w617 w626] -> w595
                  tunnel: [w616 w623] -> w590
                  frame False {
                  }
                  frame True {
                    n321 = local read "Interf.\nFrequency (Hz)"() -> (w621:dbl)
                    n322 = local read "Interf.\nAmplitude (%)"() -> (w622:dbl)
                    n323 = Divide(x=w622, y=100.0) -> (x/y=w633:dbl)
                    n324 = Multiply(x=w631, y=w633) -> (x*y=w632:dbl)
                    n325 = call <vilib>:"Sine Waveform.vi"("sampling info"=w630, "phase"=0.0, "amplitude"=w632, "frequency"=w621) -> ("error out"=w619:errorcluster, "signal out"=w624:waveform(dbl))  [unwired: 6 in]
                    n326 = Add(1:w624, 2:w627, 4:w619) -> (0:w626:waveform(dbl))  [unwired: 1 out]
                    n327 = Add(1:w624, 2:w625, 4:w619) -> (0:w623:waveform(dbl))  [unwired: 1 out]
                    n328 = Add(1:w624, 2:w629, 4:w619) -> (0:w628:waveform(dbl))  [unwired: 1 out]
                  }
                }
              }
            }
            n329 = case shown="False" "Noise" {
              tunnel: w272 -> [w283 w296]
              tunnel: w266 -> [w284 w295]
              tunnel: [w284 w294] -> w271
              tunnel: [w283 w293] -> w270
              tunnel: [w282 w292] -> w269
              tunnel: w268 -> [w282 w291]
              tunnel: w261 -> [_ w287]
              frame False {
              }
              frame True {
                # "Noise configurations"
                n330 = Bundle("#s"=w287, "#s"=w287) -> (w290:cluster{"#s":dbl, "#s":dbl})  [unwired: 1 in]
                n331 = call <vilib>:"Tones and Noise Waveform.vi"("sampling info"=w290, "offset"=0.0, "noise (rms)"="Amplitude (rms)", "tones"=T7 [{"frequency"=0.0, "amplitude"=0.0, "phase"=0.0}, {"frequency"=0.0, "amplitude"=0.0, "phase"=0.0}]) -> ("signal out"=w285:waveform(dbl))  [unwired: 6 in, 1 out]
                n332 = Add(1:w285, 2:w291) -> (0:w292:waveform(dbl))  [unwired: 1 in, 1 out]
                n333 = Add(1:w285, 2:w295) -> (0:w294:waveform(dbl))  [unwired: 1 in, 1 out]
                n334 = Add(1:w285, 2:w296) -> (0:w293:waveform(dbl))  [unwired: 1 in, 1 out]
              }
            }
          }
          frame #2 {
            # "Sinusoid > Channel 3"
            n335 = case shown="False" w660 {
              tunnel: [w696 w710] -> w670
              tunnel: [w695 w697] -> w677
              tunnel: w676 -> [_ w709]
              tunnel: [w694 w708] -> w658
              tunnel: w673 -> [_ w703]
              tunnel: w672 -> [w696 _]
              tunnel: w659 -> [w694 _]
              tunnel: w671 -> [w695 _]
              frame True {
              }
              frame False {
                w725 = 1000
                # "others phases"
                # "first phase"
                # "decimacao"
                n336 = Unbundle By Name(w703) -> ("Y"=w704:dbl[], "dt"=w705:dbl)
                n337 = Divide(x=w709, y=w725) -> (x/y=w724:dbl)
                n338 = Multiply(x=w724, y=w705) -> (x*y=w727:dbl)
                n339 = for {
                  N: w725 -> [_]
                  tunnel: w704 -> [w743]
                  tunnel: [w740] -> w728 mode=indexing
                  tunnel: w724 -> [w739]
                  i -> [w741]
                  n340 = Multiply(x=w741, y=w739) -> (x*y=w742:dbl)
                  n341 = Index Array(array=w743, index=w742) -> (element=w740:dbl)
                }
                n342 = local read "Frequency (Hz)"() -> (w718:dbl)
                n343 = local read "Pulse frequency"() -> (w714:dbl)
                n344 = Subtract(x=w718, y=50.0) -> (x-y=w717:dbl)
                n345 = Bundle By Name("Y"=w728, "dt"=w727) -> (w726:waveform(dbl))  [unwired: 1 in]
                n346 = Multiply(x=w717, y=360.0) -> (x*y=w716:dbl)
                n347 = call-poly <vilib>:"Extract Single Tone Information.vi"("time signal in"=w726) -> ("detected phase (deg)"=w722:dbl)  [unwired: 5 in, 5 out]
                n348 = Divide(x=w716, y=w714) -> (x/y=w713:dbl)
                n349 = Subtract(x=w722, y=90.0) -> (x-y=w721:dbl)
                n350 = local read "Amplitude (V)"() -> (w707:dbl)
                n351 = local read "Frequency (Hz)"() -> (w706:dbl)
                n352 = call "angle_corrector.vi"("angle"=w721) -> ("angle corrected"=w711:dbl)  [unwired: 10 in]
                "Phase (deg)" <- w711
                n353 = for {
                  N: w714 -> [_]
                  tunnel: [w732] -> w715 mode=indexing
                  tunnel: w713 -> [w736]
                  tunnel: w711 -> [w737]
                  tunnel: w707 -> [w734]
                  tunnel: [w734] -> w710 mode=indexing
                  tunnel: w706 -> [w733]
                  tunnel: [w733] -> w708 mode=indexing
                  i -> [w738]
                  n354 = Multiply(x=w736, y=w738) -> (x*y=w735:dbl)
                  n355 = Add(x=w737, y=w735) -> (x+y=w731:dbl)
                  n356 = call "angle_corrector2.vi"("angle"=w731) -> ("angle corrected"=w732:dbl)  [unwired: 10 in]
                }
                n357 = local read "phase 2"() -> (w700:dbl)
                n358 = Replace Array Subset(array=w715, new element=w711, index=0) -> (w701:dbl[])
                n359 = Multiply(x=w700, y=-2.0) -> (x*y=w699:dbl)
                n360 = Add(x=w701, y=w699) -> (x+y=w698:dbl[])
                n361 = for {
                  tunnel: w698 -> [w730] mode=indexing
                  tunnel: [w729] -> w697 mode=indexing
                  n362 = call "angle_corrector_array.vi"("angle"=w730) -> ("angle corrected"=w729:dbl)  [unwired: 10 in]
                }
              }
            }
            n363 = Unbundle By Name(w669) -> ("Y"=w665:dbl[])
            n364 = Unbundle By Name(w668) -> ("Y"=w666:dbl[])
            n365 = Unbundle By Name(w663) -> ("Y"=w661:dbl[])
            n366 = Unbundle By Name(w662) -> ("Y"=w664:dbl[])
            n367 = case shown="True" "Boolean" {
              tunnel: w676 -> [_ w689]
              tunnel: w675 -> [_ w688]
              tunnel: w661 -> [_ w687]
              tunnel: w664 -> [_ w686]
              frame False {
              }
              frame True {
                w685 = 0 ("start index (0)")
                # "First cycle visualization"
                n368 = Divide(x=w689, y=w688) -> (x/y=w692:dbl)
                n369 = To Long Integer(number=w692) -> (32bit integer=w690:i32)
                n370 = Search 1D Array(1D array=w686, element=2.95, start index (0)=w685) -> ()  [unwired: 1 out]
                n371 = Array Subset(array=w687, index=w685, length=w690) -> (→"Cycle visualization":dbl[])
              }
            }
            n372 = Build Array(w664, w661, w665, w666) -> (w674:dbl[][])
            n373 = for {
              tunnel: w658 -> [w681] mode=indexing
              shift-right: [w681] -> _
              shift-left: _ -> [w684]
              tunnel: [w680] -> w657 mode=indexing
              n374 = local read "Pulse frequency"() -> (w682:dbl)
              n375 = Subtract(x=w681, y=w684) -> (x-y=w683:dbl)
              n376 = Multiply(x=w683, y=w682) -> (x*y=w680:dbl)
            }
          }
          frame #3 {
            n377 = case shown="0, Default" w745 {
              tunnel: w744 -> [w750 w751]
              frame 0, Default {
                "rocof0" <- w750
              }
              frame 1 {
                "rocof1" <- w751
              }
            }
            n378 = case shown="1" w745 {
              tunnel: w746 -> [w752 w753]
              frame 0, Default {
                "freq0" <- w752
              }
              frame 1 {
                "freq1" <- w753
              }
            }
            n379 = case shown="1" w745 {
              tunnel: w747 -> [w754 w755]
              frame 0, Default {
                "magnitude0" <- w754
              }
              frame 1 {
                "magnitude1" <- w755
              }
            }
            n380 = case shown="0, Default" w745 {
              tunnel: w748 -> [w756 w757]
              frame 0, Default {
                "phases0" <- w756
              }
              frame 1 {
                "phases1" <- w757
              }
            }
          }
        }
        n381 = call-poly <vilib>:"DAQmx Write.vi"("task/channels in"=w72, "data"=w70, "error in"=w90) -> ("task out"=w88:refnum<k21>, "error out"=w89:errorcluster)  [unwired: 10 in, 1 out]
        n382 = node-c288() -> ()  [unwired: 5 in, 1 out]
      }
      n383 = call <vilib>:"DAQmx Stop Task.vi"("task/channels in"=w52, "error in"=w53) -> ("task out"=w59:refnum<k21>, "error out"=w38:errorcluster)  [unwired: 12 in]
      n384 = node-c288(w67) -> (→"Iteration Duration":i64)  [unwired: 6 out]
      n385 = call <vilib>:"DAQmx Clear Task.vi"("task in"=w59, "error in"=w38) -> ("error out"=w62:errorcluster)  [unwired: 13 in]
      n386 = call <vilib>:"Simple Error Handler.vi"("type of dialog (OK msg:1)"=w64, "error in (no error)"=w62) -> ()  [unwired: 3 in, 5 out]
    }
  }
  n387 = Build Array("Loop1", "Loop2") -> (w4:string[])
  n388 = call <vilib>:"Synchronize Timed Structure Starts.vi"("timed structure names"=w4, "synchronization group name"="grupo de sincronismo") -> ()  [unwired: 8 in, 2 out]
  n389 = case shown="True" "Serial communication" {
    selector: "Serial communication" -> [_ w773]
    tunnel: "Loop2" -> [_ w774]
    frame False {
    }
    frame True {
      n390 = case shown="True" w773 {
        tunnel: [_ w808] -> w791
        tunnel: [_ w800] -> w790
        frame False {
        }
        frame True {
          n391 = call-poly "VISA Configure Serial Port"("VISA resource name"="Porta", "timeout (10sec)"="timeout (ms)", "Enable Termination\nChar (T)"=FALSE ("Enable Termination\nChar (T)"), "baud rate (9600)"="baud rate (kB)", "data bits (8)"="data bits (8)", "parity (0:none)"="parity (0:none)", "stop bits (10: 1 bit)"="stop bits (10: 1 bit)", "flow control (0:none)"="flow control (0:none)") -> ("VISA resource name out"=w808:refnum<visa-resource-name>, "error out"=w800:errorcluster)  [unwired: 6 in]
        }
      }
      n392 = call-poly <vilib>:"DAQmx Create Timing Source.vi"("counter"=tag "Dev1/ctr0", "frequency"=1000.0) -> ("timing source out"=w776:string)  [unwired: 12 in, 1 out]
      n393 = Build Path(base path=path "C:/Users/Flavio-CPGEI/Dropbox/versoes 2014/Analise e calibracao/Resultados" ("file path (use dialog)"), name or relative path="File name") -> (appended path=w778:path)
      n394 = node-c288(w776, i64 0 ("Period"), 100 ("Priority"), 1 ("Processor"), w774, nitl_modes."Process missed periods, ignore original phase" ("Mode"), i64 40 ("Offset")) -> (w798:T8)  [unwired: 2 in]
      n395 = Open/Create/Replace File(file path (use dialog)=w778, operation (0:open)=T11."replace or create", access (0:read/write)=enum16{"read/write", "read-only", "write-only"}."write-only") -> (refnum out=w781:refnum<file>, error out=w782:errorcluster)  [unwired: 3 in, 1 out]
      n396 = timed-loop {
        timing: w798 -> [_]
        timing-out: [_] -> w797
        tunnel: w790 -> [w881]
        tunnel: w791 -> [w880]
        tunnel: [w879] -> w789
        tunnel: [w878] -> w788
        shift-right: [w877] -> _
        shift-left: 0 ("t") -> [w876]
        shift-right: [w839] -> _
        shift-left: 0 ("initial phase") -> [w840]
        tunnel: [w829] -> w786
        tunnel: [w828] -> w785
        tunnel: w782 -> [w827]
        tunnel: w781 -> [w826]
        i -> [w837]
        stop <- "stop" stop-if-true
        n397 = node-c288() -> (w861:errorcluster, →"Iteration Duration 2":i64)  [unwired: 1 in, 2 out]
        n398 = flat-sequence {
          tunnel: w880 -> [w922]
          tunnel: w881 -> [w923]
          tunnel: [w923] -> w857
          tunnel: [w922] -> w855
          tunnel: w876 -> [w918]
          tunnel: [w913] -> w856
          tunnel: [w936] -> w854
          tunnel: [w934] -> w853
          tunnel: [w932] -> w852
          tunnel: [w930] -> w858
          tunnel: [w942] -> w851
          tunnel: [w931] -> w859
          tunnel: [w943] -> w850
          tunnel: [w941] -> w860
          tunnel: w840 -> [w925]
          tunnel: w856 -> [w927]
          tunnel: w855 -> [w939]
          tunnel: w857 -> [w940]
          tunnel: [w928] -> w821
          tunnel: [w924] -> w816
          tunnel: w854 -> [w979]
          tunnel: w853 -> [w978]
          tunnel: w852 -> [w962]
          tunnel: w858 -> [w963]
          tunnel: w851 -> [w964]
          tunnel: w859 -> [w967]
          tunnel: w850 -> [w960]
          tunnel: w860 -> [w958]
          tunnel: [w979] -> w879
          tunnel: [w978] -> w878
          tunnel: [w966] -> w831
          tunnel: [w959] -> w832
          tunnel: [w965] -> w833
          tunnel: [w964] -> w834
          tunnel: [w961] -> w835
          tunnel: [w958] -> w836
          tunnel: [w956] -> w815
          tunnel: w821 -> [w957]
          tunnel: w816 -> [w955]
          tunnel: [w955] -> w814
          frame #0 {
            n399 = local read "Pulse frequency"() -> (w912:dbl)
            n400 = To Long Integer(number=w912) -> (32bit integer=w909:i32)
            n401 = Multiply(x=2 ("y"), y=w909) -> (x*y=w910:i32)
            n402 = Greater Or Equal?(x=w918, y=w909) -> (x >= y?=w917:bool)
            n403 = Greater Or Equal?(x=w918, y=w910) -> (x >= y?=w916:bool)
            n404 = Select(t=1, s=w917, f=0) -> (s? t:f=w914:i32)
            n405 = Wait (ms)(milliseconds to wait=u32 2) -> ()  [unwired: 1 out]
            n406 = Select(t=2, s=w916, f=w914) -> (s? t:f=w913:i32)
          }
          frame #1 {
            # "leituras"
            # "Conversor"
            n407 = VISA Flush I/O Buffer(VISA resource name=w939, error in (no error)=w940) -> (VISA resource name out=w933:refnum<visa-resource-name>, error out=w937:errorcluster)  [unwired: 1 in]
            n408 = case shown="1" w927 {
              tunnel: [w951 w952] -> w945
              frame 0, Default {
                n409 = local read "magnitude0"() -> (w951:dbl[])
              }
              frame 1 {
                n410 = local read "magnitude1"() -> (w952:dbl[])
              }
            }
            n411 = case shown="1" w927 {
              tunnel: [w953 w954] -> w946
              frame 0, Default {
                n412 = local read "phases0"() -> (w953:dbl[])
              }
              frame 1 {
                n413 = local read "phases1"() -> (w954:dbl[])
              }
            }
            n414 = case shown="0, Default" w927 {
              tunnel: [w947 w948] -> w926
              frame 0, Default {
                n415 = local read "rocof0"() -> (w947:dbl[])
              }
              frame 1 {
                n416 = local read "rocof1"() -> (w948:dbl[])
              }
            }
            n417 = case shown="0, Default" w927 {
              tunnel: [w949 w950] -> w944
              frame 0, Default {
                n418 = local read "freq0"() -> (w949:dbl[])
              }
              frame 1 {
                n419 = local read "freq1"() -> (w950:dbl[])
              }
            }
            n420 = VISA Read(VISA resource name=w933, byte count=u32 16, error in (no error)=w937) -> (VISA resource name out=w934:refnum<visa-resource-name>, read buffer=w935:string, error out=w936:errorcluster)  [unwired: 1 out]
            n421 = Index Array(array=w945, index=w925) -> (element=w943:dbl)
            n422 = Index Array(array=w926, index=w925) -> (element=w924:dbl)
            n423 = Index Array(array=w944, index=w925) -> (element=w941:dbl)
            n424 = Index Array(array=w946, index=w925) -> (element=w942:dbl)
            n425 = String To Byte Array(string=w935) -> (unsigned byte array=w929:u8[])
            n426 = call "Conversor_4dados.vi"("subarray"=w929) -> ("ROCOF"=w928:sgl, "Frequência"=w930:sgl, "Ângulo"=w931:sgl, "Módulo"=w932:sgl)  [unwired: 2 in]
          }
          frame #2 {
            # "correçoes"
            n427 = To Double Precision Float(number=w963) -> (double precision float=w968:dbl)
            n428 = To Double Precision Float(number=w957) -> (double precision float=w956:dbl)
            n429 = Square Root(x=2.0) -> (sqrt(x)=w975:dbl)
            n430 = Add(x=w968, y="Frequency\noff-set") -> (x+y=w961:dbl)
            n431 = To Double Precision Float(number=w962) -> (double precision float=w970:dbl)
            n432 = Divide(x=w960, y=w975) -> (x/y=w959:dbl)
            n433 = To Double Precision Float(number=w967) -> (double precision float=w969:dbl)
            n434 = Add(x=w969, y="Angle\noff-set") -> (x+y=w965:dbl)
            n435 = Multiply(x=w970, y="Magnitude\ncoefficient") -> (x*y=w972:dbl)
            n436 = Add(x=w972, y="Magnitude\noff-set") -> (x+y=w966:dbl)
          }
        }
        n437 = local read "Pulse frequency"() -> (w867:dbl)
        n438 = Multiply(x=w867, y=u16 2) -> (x*y=w870:dbl)
        n439 = Decrement(x=w870) -> (x-1=w869:dbl)
        n440 = Equal?(x=w869, y=w876) -> (x = y?=w866:bool)
        n441 = Increment(x=w876) -> (x+1=w865:i32)
        n442 = Select(t=0, s=w866, f=w865) -> (s? t:f=w877:i32)
        n443 = local read "Pulse frequency"() -> (w863:dbl)
        n444 = Decrement(x=w863) -> (x-1=w864:dbl)
        n445 = Equal?(x=w840, y=w864) -> (x = y?=w872:bool)
        n446 = Increment(x=w840) -> (x+1=w874:i32)
        n447 = Select(t=u16 0, s=w872, f=w874) -> (s? t:f=w839:i32)
        n448 = case shown="True" "Data save" {
          tunnel: w831 -> [_ w902]
          tunnel: w833 -> [_ w901]
          tunnel: w835 -> [_ w899]
          tunnel: w836 -> [_ w898]
          tunnel: w837 -> [_ w893]
          tunnel: w834 -> [_ w900]
          tunnel: w832 -> [_ w895]
          tunnel: [_ w892] -> w830
          tunnel: w815 -> [_ w891]
          tunnel: w814 -> [_ w890]
          frame False {
          }
          frame True {
            w894 = "\t"
            n449 = feedback #14(w893) -> (w897:i32)
            n450 = feedback-in #14(w897) -> ()
            n451 = Subtract(x=w893, y=w897) -> (x-y=w896:i32)
            n452 = Format Into String(w896, w894, w902, w894, w895, w894, w901, w894, w900, w894, w899, w894, w898, w894, w891, w894, w890, "\r\n") -> (resulting string=w892:string)  [unwired: 3 in, 1 out]
          }
        }
        n453 = Initialize Array(w831, 1 ("dimension size")) -> (w818:dbl[])
        "Voltage measured" <- w818
        n454 = Initialize Array(w832, 1 ("dimension size")) -> (w819:dbl[])
        "Voltage reference" <- w819
        n455 = Initialize Array(w833, 1 ("dimension size")) -> (w809:dbl[])
        "Angle measured" <- w809
        n456 = Initialize Array(w834, 1 ("dimension size")) -> (w810:dbl[])
        "Angle reference" <- w810
        n457 = Write to Text File(file (use dialog)=w826, text=w830, error in=w827) -> (refnum out=w828:refnum<file>, error out=w829:errorcluster)  [unwired: 1 in, 1 out]
        n458 = Initialize Array(w815, 1 ("dimension size")) -> (w817:dbl[])
        "ROCOF measured" <- w817
        n459 = Initialize Array(w814, 1 ("dimension size")) -> (w822:dbl[])
        "ROCOF reference" <- w822
        n460 = Initialize Array(w835, 1 ("dimension size")) -> (w811:dbl[])
        "Frequency measured" <- w811
        n461 = Initialize Array(w836, 1 ("dimension size")) -> (w812:dbl[])
        "Frequency reference" <- w812
        n462 = case shown="True" "?" {
          tunnel: w818 -> [_ w989]
          tunnel: w819 -> [_ w988]
          frame False {
          }
          frame True {
            n463 = Build Array(w989, w988) -> (w991:dbl[][])
            n464 = Transpose 2D Array(2D array=w991) -> (transposed array=→"Magnitude measures (V)":dbl[][])
          }
        }
        n465 = case shown="True" "?" {
          tunnel: w810 -> [_ w984]
          tunnel: w809 -> [_ w985]
          frame False {
          }
          frame True {
            n466 = Build Array(w985, w984) -> (w987:dbl[][])
            n467 = Transpose 2D Array(2D array=w987) -> (transposed array=→"Phase measures (º)":dbl[][])
          }
        }
        n468 = case shown="True" "?" {
          tunnel: w817 -> [_ w886]
          tunnel: w822 -> [_ w885]
          frame False {
          }
          frame True {
            n469 = Build Array(w886, w885) -> (w887:dbl[][])
            n470 = Transpose 2D Array(2D array=w887) -> (transposed array=→"ROCOF (Hz/s)":dbl[][])
          }
        }
        n471 = case shown="True" "?" {
          tunnel: w812 -> [_ w982]
          tunnel: w811 -> [_ w981]
          frame False {
          }
          frame True {
            n472 = Build Array(w981, w982) -> (w983:dbl[][])
            n473 = Transpose 2D Array(2D array=w983) -> (transposed array=→"Frequency measures (Hz)":dbl[][])
          }
        }
        n474 = case shown="True" "Boolean 3" {
          tunnel: w819 -> [_ w904]
          tunnel: w818 -> [_ w906]
          tunnel: w809 -> [_ w905]
          tunnel: w810 -> [_ w903]
          frame False {
          }
          frame True {
            n475 = call-poly <vilib>:"Plot Helper.vi"("radius vector"=w906, "theta vector"=w905) -> ("2D Plot Class Obj Array out"=w907:refnum<class "2D Plot Datatype.lvclass">[])  [unwired: 2 in, 7 out]
            n476 = call-poly <vilib>:"Plot Helper.vi"("radius vector"=w904, "theta vector"=w903, "2D Plot Class Obj Array in"=w907) -> ("2D Plot Class Obj Array out"=→"Phasors visualization":refnum<class "2D Plot Datatype.lvclass">[])  [unwired: 1 in, 7 out]
          }
        }
        n477 = case shown="True" "?" {
          tunnel: w810 -> [_ w884]
          tunnel: w809 -> [_ w883]
          frame False {
          }
          frame True {
            n478 = Subtract(x=w884, y=w883) -> (x-y=→"Phase measures (º) 2":dbl[])
          }
        }
        n479 = node-c288(w861) -> ()  [unwired: 1 out]
      }
      n480 = node-c288(w797) -> ()  [unwired: 1 out]
      n481 = Close File(refnum=w785, error in=w786) -> ()  [unwired: 2 out]
      n482 = VISA Close(VISA resource name=w788, error in (no error)=w789) -> ()  [unwired: 1 out]
    }
  }
  n483 = case shown="True" FALSE {
    frame False {
    }
    frame True {
      n484 = while {
        stop <- FALSE stop-if-true
        n485 = case shown="\"Real-Time Data\"" "Tab Control" {
          frame "Communication", Default {
          }
          frame "Real-Time Data" {
            n486 = local read "Pulse frequency"() -> (w1012:dbl)
            n487 = Initialize Array(0.0 ("element"), w1012) -> (w1011:dbl[])
            "initialized array" <- w1011
            n488 = while {
              shift-right: [w1051] -> _
              shift-left: 0 -> [w1028]
              tunnel: w1012 -> [w1050]
              tunnel: w1011 -> [w1025]
              stop <- w1041 stop-if-true
              # "Escrevem nos controles da  aba principal"
              # "Controles da aba Real-Time Data"
              # "Indicadores da aba Real-Time Data"
              n489 = local read "Phase (deg)"() -> (→"Phase (degrees) 2":dbl)
              n490 = Wait (ms)(milliseconds to wait=u32 30) -> ()  [unwired: 1 out]
              n491 = local read "ROCOF measured"() -> (w1026:dbl[])
              n492 = local read "ROCOF reference"() -> (w1027:dbl[])
              n493 = local read "Frequency reference"() -> (w1034:dbl[])
              n494 = local read "Voltage measured"() -> (w1022:dbl[])
              n495 = local read "Frequency measured"() -> (w1033:dbl[])
              n496 = local read "Angle measured"() -> (w1031:dbl[])
              n497 = local read "Angle reference"() -> (w1032:dbl[])
              n498 = local read "Voltage reference"() -> (w1021:dbl[])
              n499 = Equal?(x=w1050, y=w1028) -> (x = y?=w1042:bool)
              n500 = Increment(x=w1028) -> (x+1=w1053:i32)
              n501 = feedback #15(w1025) -> (w1059:dbl[])
              n502 = Replace Array Subset(array=w1059, new element=w1021, index=w1028) -> (w1045:dbl[])
              n503 = feedback-in #15(w1045) -> ()
              n504 = feedback #16(w1025) -> (w1058:dbl[])
              n505 = Replace Array Subset(array=w1058, new element=w1022, index=w1028) -> (w1046:dbl[])
              n506 = feedback-in #16(w1046) -> ()
              n507 = feedback #17(w1025) -> (w1055:dbl[])
              n508 = Replace Array Subset(array=w1055, new element=w1033, index=w1028) -> (w1043:dbl[])
              n509 = feedback-in #17(w1043) -> ()
              n510 = feedback #18(w1025) -> (w1054:dbl[])
              n511 = Replace Array Subset(array=w1054, new element=w1034, index=w1028) -> (w1044:dbl[])
              n512 = feedback-in #18(w1044) -> ()
              n513 = feedback #19(w1025) -> (w1057:dbl[])
              n514 = Replace Array Subset(array=w1057, new element=w1031, index=w1028) -> (w1047:dbl[])
              n515 = feedback-in #19(w1047) -> ()
              n516 = feedback #20(w1025) -> (w1056:dbl[])
              n517 = Replace Array Subset(array=w1056, new element=w1032, index=w1028) -> (w1048:dbl[])
              n518 = feedback-in #20(w1048) -> ()
              n519 = feedback #21(w1025) -> (w1030:dbl[])
              n520 = Replace Array Subset(array=w1030, new element=w1026, index=w1028) -> (w1024:dbl[])
              n521 = feedback-in #21(w1024) -> ()
              n522 = feedback #22(w1025) -> (w1029:dbl[])
              n523 = Replace Array Subset(array=w1029, new element=w1027, index=w1028) -> (w1023:dbl[])
              n524 = feedback-in #22(w1023) -> ()
              n525 = Select(t=0, s=w1042, f=w1053) -> (s? t:f=w1051:i32)
              n526 = case shown="True" w1042 {
                selector: w1042 -> [_ w1071]
                tunnel: w1048 -> [_ w1087]
                tunnel: w1047 -> [_ w1086]
                tunnel: w1046 -> [_ w1061]
                tunnel: w1045 -> [_ w1070]
                tunnel: w1044 -> [_ w1081]
                tunnel: w1043 -> [_ w1080]
                tunnel: [FALSE w1071] -> w1041
                tunnel: w1024 -> [_ w1066]
                tunnel: w1023 -> [_ w1065]
                frame False {
                }
                frame True {
                  n527 = call "Statistical measure - basics - 4.vi"("Data measured"=w1066, "Data reference"=w1065) -> ("Statistcs"=w1064:T12)  [unwired: 12 in, 1 out]
                  n528 = Add Array Elements(numeric array=w1061) -> (sum=w1069:dbl)
                  n529 = Array Size(array=w1061) -> (size(s)=w1068:i32)
                  n530 = call "Statistical measure - basics percentual - 1.vi"("Data measured"=w1070, "Data reference"=w1061) -> ("Statistcs"=w1082:T12)  [unwired: 12 in, 1 out]
                  n531 = call "Statistical measure - basics - 1.vi"("Data measured"=w1086, "Data reference"=w1087) -> ("Statistcs"=w1089:T12)  [unwired: 12 in, 1 out]
                  n532 = call "Statistical measure - basics - 3.vi"("Data measured"=w1080, "Data reference"=w1081) -> ("Statistcs"=w1079:T12)  [unwired: 12 in, 1 out]
                  n533 = call "TVE.vi"("Angle reference"=w1087, "Angle measured"=w1086, "Voltage reference"=w1061, "Voltage measured"=w1070) -> ("Array"=w1084:dbl[])
                  n534 = local read "initialized array"() -> (w1085:dbl[])
                  n535 = Unbundle By Name(w1064) -> ("max dev"=→"max rocof":dbl, "mean dev"=→"mean rocof":dbl)
                  n536 = Unbundle By Name(w1082) -> ("max dev"=→"max magnitude":dbl, "mean dev"=→"mean dev":dbl)
                  n537 = Divide(x=w1069, y=w1068) -> (x/y=→"Media":dbl)
                  n538 = Unbundle By Name(w1089) -> ("max dev"=→"max phase":dbl, "mean dev"=→"mean phase":dbl)
                  n539 = Unbundle By Name(w1079) -> ("max dev"=→"max freq":dbl, "mean dev"=→"mean freq":dbl)
                  n540 = call "Statistical measure - basics - 2.vi"("Data measured"=w1084, "Data reference"=w1085) -> ("Statistcs"=w1083:T12)  [unwired: 12 in, 1 out]
                  n541 = Unbundle By Name(w1083) -> ("max dev"=→"max tve":dbl, "mean dev"=→"mean tve":dbl)
                }
              }
              n542 = local write "Amplitude (%)"("Amp. (%) 2") -> ()
              n543 = local write "Interf.\nFrequency (Hz)"("Interf. Frequency 2") -> ()
              n544 = local write "Interf.\nAmplitude (%)"("amplitude") -> ()
              n545 = local write "Interference"("Interference 2") -> ()
              n546 = local write "Order"("Order 2") -> ()
              n547 = local write "Harmonics"("Harmonics 2") -> ()
              n548 = local write "Offset"("Offset 2") -> ()
              n549 = local write "Phase"("Phase 2") -> ()
              n550 = local write "Amplitude"("Amplitude 2") -> ()
              n551 = local write "Frequency"("Frequency 2") -> ()
              n552 = local write "reset\nphase?"("reset signal 2") -> ()
            }
          }
          frame "Measure statistics" {
          }
        }
        n553 = Wait (ms)(milliseconds to wait=u32 1000) -> ()  [unwired: 1 out]
      }
    }
  }
